vi "Main.vi"() -> ()   [LabVIEW 2013]
uses:
  <vilib>/event_ctls.llb/eventvkey.ctl
  skripte/Element 1.ctl
  Global_Not-Aus.vi
  <vilib>/Utility/file.llb/Read From Spreadsheet File (DBL).vi
  Global_Start_Stop_Einzelschritt.vi
  <vilib>/Utility/file.llb/Write To Spreadsheet File (DBL).vi
  <vilib>/Utility/file.llb/Read From Spreadsheet File (string).vi
  <vilib>/Utility/file.llb/Write To Spreadsheet File (string).vi
  <vilib>/Instr/_visa.llb/VISA Configure Serial Port (Instr).vi
panel:
  out "temp":string
  in  "stop handover":bool
  in  "Polplan":string[](array[string])
  in  "load polplan":bool
  in  "Second head On/Off":bool
  in  "path polplan":path
  in  "distance measure mode":string(combo)="ED33"
  in  "start auto write":bool
  out "key stm 2":string
  in  "baud rate (9600) 4":u32=921600 caption="Baudrate (9600)"
  in  "baud rate (9600) 3":u32=19200 caption="Baudrate (9600)"
  in  "string to write 2":string="?MEAS\r" caption="Zu schreibender String"
  out "read string 8":string caption="Gelesener String"
  out "read string 7":string caption="Gelesener String"
  in  "delay before read (ms) 7":u32=300 caption="Verzögerung vor dem Lesen (ms)"
  out "Mess Zähler":dbl
  in  "Boolesch1 25":bool
  in  "Pfad 2":path
  in  "path Selection":T1(ring)
  in  "Boolesch1 24":bool
  in  "Boolesch1 23":bool
  in  "Boolesch1 22":bool
  in  "Boolesch1 21":bool
  in  "Boolesch1 20":bool
  in  "Boolesch1 19":bool
  in  "Boolesch1 18":bool
  in  "Boolesch1 17":bool
  in  "Boolesch1 16":bool
  in  "Boolesch1":bool
  in  "Boolesch1 15":bool
  in  "Boolesch1 14":bool
  in  "Boolesch1 13":bool
  in  "Boolesch1":bool
  in  "Boolesch1 12":bool
  in  "Boolesch1 11":bool
  in  "Boolesch1 3":bool
  in  "Boolesch1 2":bool
  in  "Boolesch1":bool
  in  "Boolesch1":bool
  in  "Pfad 20":path
  in  "Pfad 19":path
  in  "Pfad 18":path
  in  "Pfad 17":path
  in  "Pfad 16":path
  in  "Pfad 15":path
  in  "Pfad 14":path
  in  "Pfad 13":path
  in  "Pfad 12":path
  in  "Pfad 11":path
  in  "Pfad 10":path
  in  "Pfad 9":path
  in  "Pfad 8":path
  in  "Pfad 7":path
  in  "Pfad 6":path
  in  "Pfad 5":path
  in  "Pfad 4":path
  in  "Pfad2":path
  in  "Pfad 0":path
  out "Messsensor":string
  out "key stm 5":string
  out "key stm 4":string
  out "key stm 3":string
  in  "baud rate 6":u32=921600 caption="Baudrate"
  in  "data bits 6":u16=8 caption="Datenbits" min=5 max=8 step=1
  in  "parity 6":u16(ring) caption="Parität" items=["Keine", "Ungerade", "Gerade", "Mark", "Space"]
  in  "stop bits 6":u16(ring)=10 caption="Stoppbits" items=["1.0"=10, "1.5"=15, "2.0"=20]
  in  "flow control 6":u16(ring) caption="Ablaufsteuerung" items=["Keine"=0, "XON/XOFF"=1, "RTS/CTS"=2, "DTR/DSR"=4]
  in  "baud rate (9600) 2":u32=115200 caption="Baudrate (9600)"
  in  "delay before read (ms) 6":u32=100 caption="Verzögerung vor dem Lesen (ms)"
  in  "write ED33":string="?\r" caption="Remote_Modus"
  out "bytes read 6":u32 caption="Gelesene Bytes"
  out "read string 6":string caption="Gelesener String2"
  in  "write KMT":string="o\r" caption="Remote_Modus"
  out "read string 5":string caption="Gelesener String"
  in  "Start ED33 schreiben":bool
  out "read string 4":string caption="Gelesener String"
  out "bytes read 5":u32 caption="Gelesene Bytes"
  in  "write 10":string="Z\r" caption="Remote_Modus"
  in  "delay before read (ms) 5":u32=100 caption="Verzögerung vor dem Lesen (ms)"
  in  "write 9":bool=TRUE caption="Schreiben"
  in  "flow control 5":u16(ring) caption="Ablaufsteuerung" items=["Keine"=0, "XON/XOFF"=1, "RTS/CTS"=2, "DTR/DSR"=4]
  in  "stop bits 5":u16(ring)=10 caption="Stoppbits" items=["1.0"=10, "1.5"=15, "2.0"=20]
  in  "parity 5":u16(ring) caption="Parität" items=["Keine", "Ungerade", "Gerade", "Mark", "Space"]
  in  "data bits 5":u16=8 caption="Datenbits" min=5 max=8 step=1
  in  "VISA-Referenz (Eingang) 3":refnum<visa-resource-name>="COM7" caption="VISA-Ressourcenname"
  in  "baud rate 5":u32=921600 caption="Baudrate"
  out "bytes read 4":u32 caption="Gelesene Bytes"
  in  "write9":string="Z\r" caption="Remote_Modus"
  in  "delay before read (ms) 4":u32=100 caption="Verzögerung vor dem Lesen (ms)"
  in  "write 8":bool=TRUE caption="Schreiben"
  in  "flow control 4":u16(ring) caption="Ablaufsteuerung" items=["Keine"=0, "XON/XOFF"=1, "RTS/CTS"=2, "DTR/DSR"=4]
  in  "stop bits 4":u16(ring)=10 caption="Stoppbits" items=["1.0"=10, "1.5"=15, "2.0"=20]
  in  "parity 4":u16(ring) caption="Parität" items=["Keine", "Ungerade", "Gerade", "Mark", "Space"]
  in  "data bits 4":u16=8 caption="Datenbits" min=5 max=8 step=1
  in  "VISA-Referenz (Eingang) 2":refnum<visa-resource-name>="COM7" caption="VISA-Ressourcenname"
  in  "baud rate 4":u32=921600 caption="Baudrate"
  out "Position Y ED33 2":string
  out "bytes read 3":u32 caption="Gelesene Bytes"
  in  "write 7":string="?\r" caption="Remote_Modus"
  in  "delay before read (ms) 3":u32=100 caption="Verzögerung vor dem Lesen (ms)"
  in  "write 6":bool=TRUE caption="Schreiben"
  in  "flow control 3":u16(ring) caption="Ablaufsteuerung" items=["Keine"=0, "XON/XOFF"=1, "RTS/CTS"=2, "DTR/DSR"=4]
  in  "stop bits 3":u16(ring)=10 caption="Stoppbits" items=["1.0"=10, "1.5"=15, "2.0"=20]
  in  "parity 3":u16(ring) caption="Parität" items=["Keine", "Ungerade", "Gerade", "Mark", "Space"]
  in  "data bits 3":u16=8 caption="Datenbits" min=5 max=8 step=1
  in  "VISA-Referenz (Eingang)":refnum<visa-resource-name>="COM7" caption="VISA-Ressourcenname"
  in  "baud rate 3":u32=921600 caption="Baudrate"
  out "Position Y ED33":string
  out "read string 3":string caption="Gelesener String"
  out "bytes read 2":u32 caption="Gelesene Bytes"
  in  "delay before read (ms) 2":u32=100 caption="Verzögerung vor dem Lesen (ms)"
  in  "write 4":bool=TRUE caption="Schreiben"
  in  "flow control 2":u16(ring) caption="Ablaufsteuerung" items=["Keine"=0, "XON/XOFF"=1, "RTS/CTS"=2, "DTR/DSR"=4]
  in  "stop bits 2":u16(ring)=10 caption="Stoppbits" items=["1.0"=10, "1.5"=15, "2.0"=20]
  in  "parity 2":u16(ring) caption="Parität" items=["Keine", "Ungerade", "Gerade", "Mark", "Space"]
  in  "data bits 2":u16=8 caption="Datenbits" min=5 max=8 step=1
  in  "baud rate 2":u32=921600 caption="Baudrate"
  in  "delay before read (ms)":u32=100 caption="Verzögerung vor dem Lesen (ms)"
  in  "write 3":string="?\r" caption="Remote_Modus"
  out "bytes read":u32 caption="Gelesene Bytes"
  out "Serial Settings:Number of Bytes at Serial Port":u32
  out "read string 2":string caption="Gelesener String2"
  in  "write 2":string="os\r" caption="Remote_Modus"
  out "read string":string caption="Gelesener String"
  in  "baud rate (9600)":u32=115200 caption="Baudrate (9600)"
  in  "flow control":u16(ring) caption="Ablaufsteuerung" items=["Keine"=0, "XON/XOFF"=1, "RTS/CTS"=2, "DTR/DSR"=4]
  in  "stop bits":u16(ring)=10 caption="Stoppbits" items=["1.0"=10, "1.5"=15, "2.0"=20]
  in  "parity":u16(ring) caption="Parität" items=["Keine", "Ungerade", "Gerade", "Mark", "Space"]
  in  "data bits":u16=8 caption="Datenbits" min=5 max=8 step=1
  in  "baud rate":u32=921600 caption="Baudrate"
  in  "Normal Betrieb":bool
  in  "Standard memory":T2={"mm Xmin "=0.0, "mm Xmax "=100.0, " mm Ymin "=0.0, "mm Ymax "=267.9, " mm Zmin"=0.0, "mm Zmax "=108.0, "Schritte oder mm Umin (0)"=0.0, "Schritte oder mm Umax (0)"=0.0, "Schritte oder mm Cmin (0)"=0.0, "Schritte oder mm Cmax (0)"=0.0, "Schritte oder mm Amin (0)"=0.0, "Schritte oder mm Amax (0)"=0.0, "Schritte oder mm Bmin (0)"=0.0, "Schritte oder mm Bmax (0)"=0.0}
  in  "save reference kmt":bool
  in  "go to reference kmt":bool
  in  "set reference KMT":bool
  out "Referenz KMT":dbl[](array[numeric])
  out "current sequence":string[](array[string])
  in  "sequence active?":bool
  in  "clear sequence":bool
  in  "Load sequence":bool
  in  "Pfad 1":path
  out "sequence":string[][](array[string])
  in  "save reference head":bool
  in  "go to reference head":bool
  in  "set reference head":bool
  out "Reference Write head":dbl[](array[numeric])
  out "KMT Output":string
  out "STM run":dbl
  out "Write head Output":string
  in  "Power Supply Init":T3(tab)
  in  "go relative":T4
  in  "straight absolute":bool
  in  "go to exchange position":bool
  in  "read":bool
  in  "set speed btn":bool
  in  "set speed":dbl caption="[mm/s]"
  in  "go straight relative":bool
  in  "magnetization set":bool
  in  "magnetization":u16(ring) items=["off", "positive", "negative"]
  in  "command list":string(combo)
  in  "manual control OK":bool
  in  "coordinates":dbl[](array[numeric])
  in  "Absolute":bool
  out "KMT read":bool
  in  "Distances":T5
  in  "Direction 2":T6 {"Richtung Z (vEw)" items=["vom Endschalter weg", "zum Endschalter hin"]; "Richtung Y (vEw)" items=["vom Endschalter weg", "zum Endschalter hin"]; "Richtung X (vEw)" items=["vom Endschalter weg", "zum Endschalter hin"]}
  out "Measurement start value":T7
  in  "Movement":dbl[](array[numeric])
  out "ED33reading":bool
  out "GAUS read":bool
  in  "p10":dbl[](array[numeric])
  in  "p9":dbl[](array[numeric])
  in  "p8":dbl[](array[numeric])
  in  "p7":dbl[](array[numeric])
  in  "p6":dbl[](array[numeric])
  in  "p5":dbl[](array[numeric])
  in  "p4":dbl[](array[numeric])
  in  "p3":dbl[](array[numeric])
  in  "p2":dbl[](array[numeric])
  in  "Enum":T8(ring)
  in  "p1":dbl[](array[numeric])
  in  "speichern":bool
  in  "Batch field memory":path=path "Y:/01_Projekte/EPN93031_Schreibplatz/8_Konstruktionsunterlagen/8.5_Software/KOSY Steuerung LabVIEW/Batch_position1" caption="Dateipfad (Dialog, wenn leer)"
  in  "Als Standart":bool
  in  "bo to batch":bool
  in  "Enum 2":T9(ring)
  out "sensor log":string[][](table)
  in  "clear sensor log":bool
  in  "sequence path":path
  in  "open Log":bool
  in  "save log":bool
  out "XY Graph":cluster{"Y":dbl[], "Y":dbl[]}[](graph) caption="XY-Graph"
  in  "Plot":u16(ring)=6 items=["Sinus1"=5, "Cosinus1"=6, "Sinus2"=7, "Cosinus2"=8]
  out "Array":string[](array[string])
  in  "sensor run constant read":bool
  out "error IO":errorcluster caption="Error In"
  out "log":string
  out "movement":T10={"Achsen-Wahl (X)"=36, "Richtung (vEw)"=0, "Geschwindigkeit\nin mm/s (5)[0,025-20]"=5.0, "IV6"=FALSE} {"Richtung (vEw)" items=["vom Endschalter weg", "zum Endschalter hin"]; "Geschwindigkeit\nin mm/s (5)[0,025-20]" min=0.025 max=20; "Achsen-Wahl (X)" items=["X-Achse"=36, "Y-Achse"=37, "Z-Achse"=38, "U-Achse"=63]}
  out "key":T12
  in  "Anwenden":bool
  in  "Set as new standard":bool
  in  "Standartwiderherstellen Bereiche":bool
  out "Power supply init":string[](array[string])
  in  "Bereiche  X,Y,Z":T2={"mm Xmin "=0.0, "mm Xmax "=100.0, " mm Ymin "=0.0, "mm Ymax "=267.9, " mm Zmin"=0.0, "mm Zmax "=108.0, "Schritte oder mm Umin (0)"=0.0, "Schritte oder mm Umax (0)"=0.0, "Schritte oder mm Cmin (0)"=0.0, "Schritte oder mm Cmax (0)"=0.0, "Schritte oder mm Amin (0)"=0.0, "Schritte oder mm Amax (0)"=0.0, "Schritte oder mm Bmin (0)"=0.0, "Schritte oder mm Bmax (0)"=0.0}
  in  "Choose file spaces":path=path "Y:/01_Projekte/EPN93031_Schreibplatz/8_Konstruktionsunterlagen/8.5_Software/KOSY Steuerung LabVIEW/Bereichsref"
  in  "Port KOSY":refnum<visa-resource-name>="COM2"
  in  "Port ED32i":refnum<visa-resource-name>="COM8"
  in  "Port ED33":refnum<visa-resource-name>="COM7"
  in  "Port Write head":refnum<visa-resource-name>="COM4"
  in  "Port Netzteil":refnum<visa-resource-name>="COM3" caption="Port Power Supply"
  in  "KMT Port":refnum<visa-resource-name>="COM11" caption="Port KMT"
  in  "GAUS Port":refnum<visa-resource-name>="COM5" caption="Port GAUS"
  in  "GAUS read strart 2":bool
  in  "Save as text":bool
  out "Attached Array":string[][](array[string])
  in  "ED 33 Start":bool
  in  "write 5":string="z\r" caption="ED33 reset"
  in  "KMT read start":bool
  in  "Path to save txt files":path=path "Y:/01_Projekte/EPN93031_Schreibplatz/8_Konstruktionsunterlagen/8.5_Software/KOSY Steuerung LabVIEW/Messdaten Speicher"
  in  "stop program":bool
  out "moving":bool
  out "Stopped":bool
  out "current coordinates":T7
  out "speed":dbl(knob) scale=0.0..20.0
  out "key stm":string
  out "cancel state":string
  # "adress  ADR 00"
  # "remote mode"
  # "Set voltage to 10 V"
  # "Set  current to 1 A"
  # "adress  ADR 01"
  # "remote mode"
  # "Set voltage to 10 V"
  # "Set  current to 1 A"
  # "Sensors"
  # "power supply"
  # "KOSY"
types:
  T1 = enum16{"0", "1", "2", "3", "4", "5", "6", "7", "8", "9", "10", "11", "12", "13", "14", "15", "16", "17", "18", "19", "20", ""}
  T2 = cluster{"mm Xmin ":sgl, "mm Xmax ":sgl, " mm Ymin ":sgl, "mm Ymax ":sgl, " mm Zmin":sgl, "mm Zmax ":sgl, "Schritte oder mm Umin (0)":sgl, "Schritte oder mm Umax (0)":sgl, "Schritte oder mm Cmin (0)":sgl, "Schritte oder mm Cmax (0)":sgl, "Schritte oder mm Amin (0)":sgl, "Schritte oder mm Amax (0)":sgl, "Schritte oder mm Bmin (0)":sgl, "Schritte oder mm Bmax (0)":sgl}
  T3 = enum32{"manual control", "Polstreifen", "MeasuringField", "BatchField", "sensor log", "Sensorfahrt", "debug", "Info", "settings", "sensor log 2"}
  T4 = typedef "Element 1.ctl" = bool
  T5 = cluster{"X-Abstand (0)":sgl, "Y-Abstand (0)":sgl, "Z-Abstand (0)":sgl}
  T6 = cluster{"Richtung X (vEw)":u16, "Richtung Y (vEw)":u16, "Richtung Z (vEw)":u16}
  T7 = cluster{"steps x":dbl, "steps y":dbl, "steps z":dbl, "steps u":dbl, "steps c":dbl, "steps a":dbl, "steps b":dbl}
  T8 = enum16{"Position 1", "Position 2", "Position 3", "Position 4", "Position 5", "Position 6", "Position 7", "Position 8", "Position 9", "Position 10"}
  T9 = enum16{"p1", "p2", "p3", "p4", "p5", "p6", "p7", "p8", "p9", "p10"}
  T10 = cluster{"Achsen-Wahl (X)":u8, "Richtung (vEw)":u8, "Geschwindigkeit\nin mm/s (5)[0,025-20]":sgl, "IV6":bool}
  T11 = typedef "eventvkey.ctl" = enum16{"ASCII", "Enter", "Return", "Shift", "Ctrl", "Alt", "Cmd", "Opt", "Caps", "NumLock", "Clear", "Break", "Up", "Down", "Left", "Right", "Insert", "Delete", "Home", "End", "PageUp", "PageDown", "Escape", "Help", "Pause", "ScrollLock", "F1", "F2", "F3", "F4", "F5", "F6", "F7", "F8", "F9", "F10", "F11", "F12", "F13", "F14", "F15", "F16", "F17", "F18", "F19", "F20", "F21", "F22", "F23", "F24", "Play", "VolumeUp", "VolumeDown", "Mute", "Two Byte Char"}
  T12 = cluster{"laufende Nummer":i16, "Vkey":T11, "Taste":i32}
  T13 = enum16{"vom Endschalter weg", "zum Endschalter hin"}
  T14 = enum16{"zum Endschalter hin", "vom Endschalter weg"}
  T15 = cluster{"[0]":sgl, "[1]":sgl, "[2]":sgl, "[3]":sgl, "[4]":sgl, "[5]":sgl, "[6]":sgl, "[7]":sgl, "[8]":sgl, "[9]":sgl, "[10]":sgl, "[11]":sgl, "[12]":sgl, "[13]":sgl}
  T16 = cluster{"Schritte X":sgl, "Schritte Y":sgl, "Schritte Z":sgl, "Schritte U":sgl, "Schritte C":sgl, "Schritte A":sgl, "Schritte B":sgl}
  T17 = cluster{"Element":dbl, "Element":dbl, "Element":dbl}
  T18 = cluster{"coordinates[0]":dbl, "coordinates[1]":dbl, "coordinates[2]":dbl, "coordinates[3]":dbl, "coordinates[4]":dbl, "coordinates[5]":dbl, "coordinates[6]":dbl, "coordinates[7]":dbl, "coordinates[8]":dbl}
  T19 = cluster{u16, enum16{"vom Endschalter weg", "zum Endschalter hin"}, enum16{"vom Endschalter weg", "zum Endschalter hin"}}
  T20 = cluster{"coordinates[0]":dbl, "coordinates[1]":dbl, "coordinates[2]":dbl}
  T21 = cluster{"[0]":dbl, "[1]":dbl, "[2]":dbl, "[3]":dbl, "[4]":dbl, "[5]":dbl, "[6]":dbl, "[7]":dbl, "[8]":dbl}
  T22 = cluster{"Movement[0]":dbl, "Movement[1]":dbl, "Movement[2]":dbl, "Movement[3]":dbl, "Movement[4]":dbl, "Movement[5]":dbl, "Movement[6]":dbl, "Movement[7]":dbl, "Movement[8]":dbl}
  T23 = cluster{"Movement[0]":dbl, "Movement[1]":dbl, "Movement[2]":dbl, "X-Abstand (0)":sgl, "Y-Abstand (0)":sgl, "Z-Abstand (0)":sgl, "Movement[6]":dbl, "Movement[7]":dbl, "Movement[8]":dbl}
  T24 = cluster{"[0]":string, "[1]":string, "[2]":string, "[3]":string, "[4]":string, "[5]":string, "[6]":string, "[7]":string, "[8]":string}
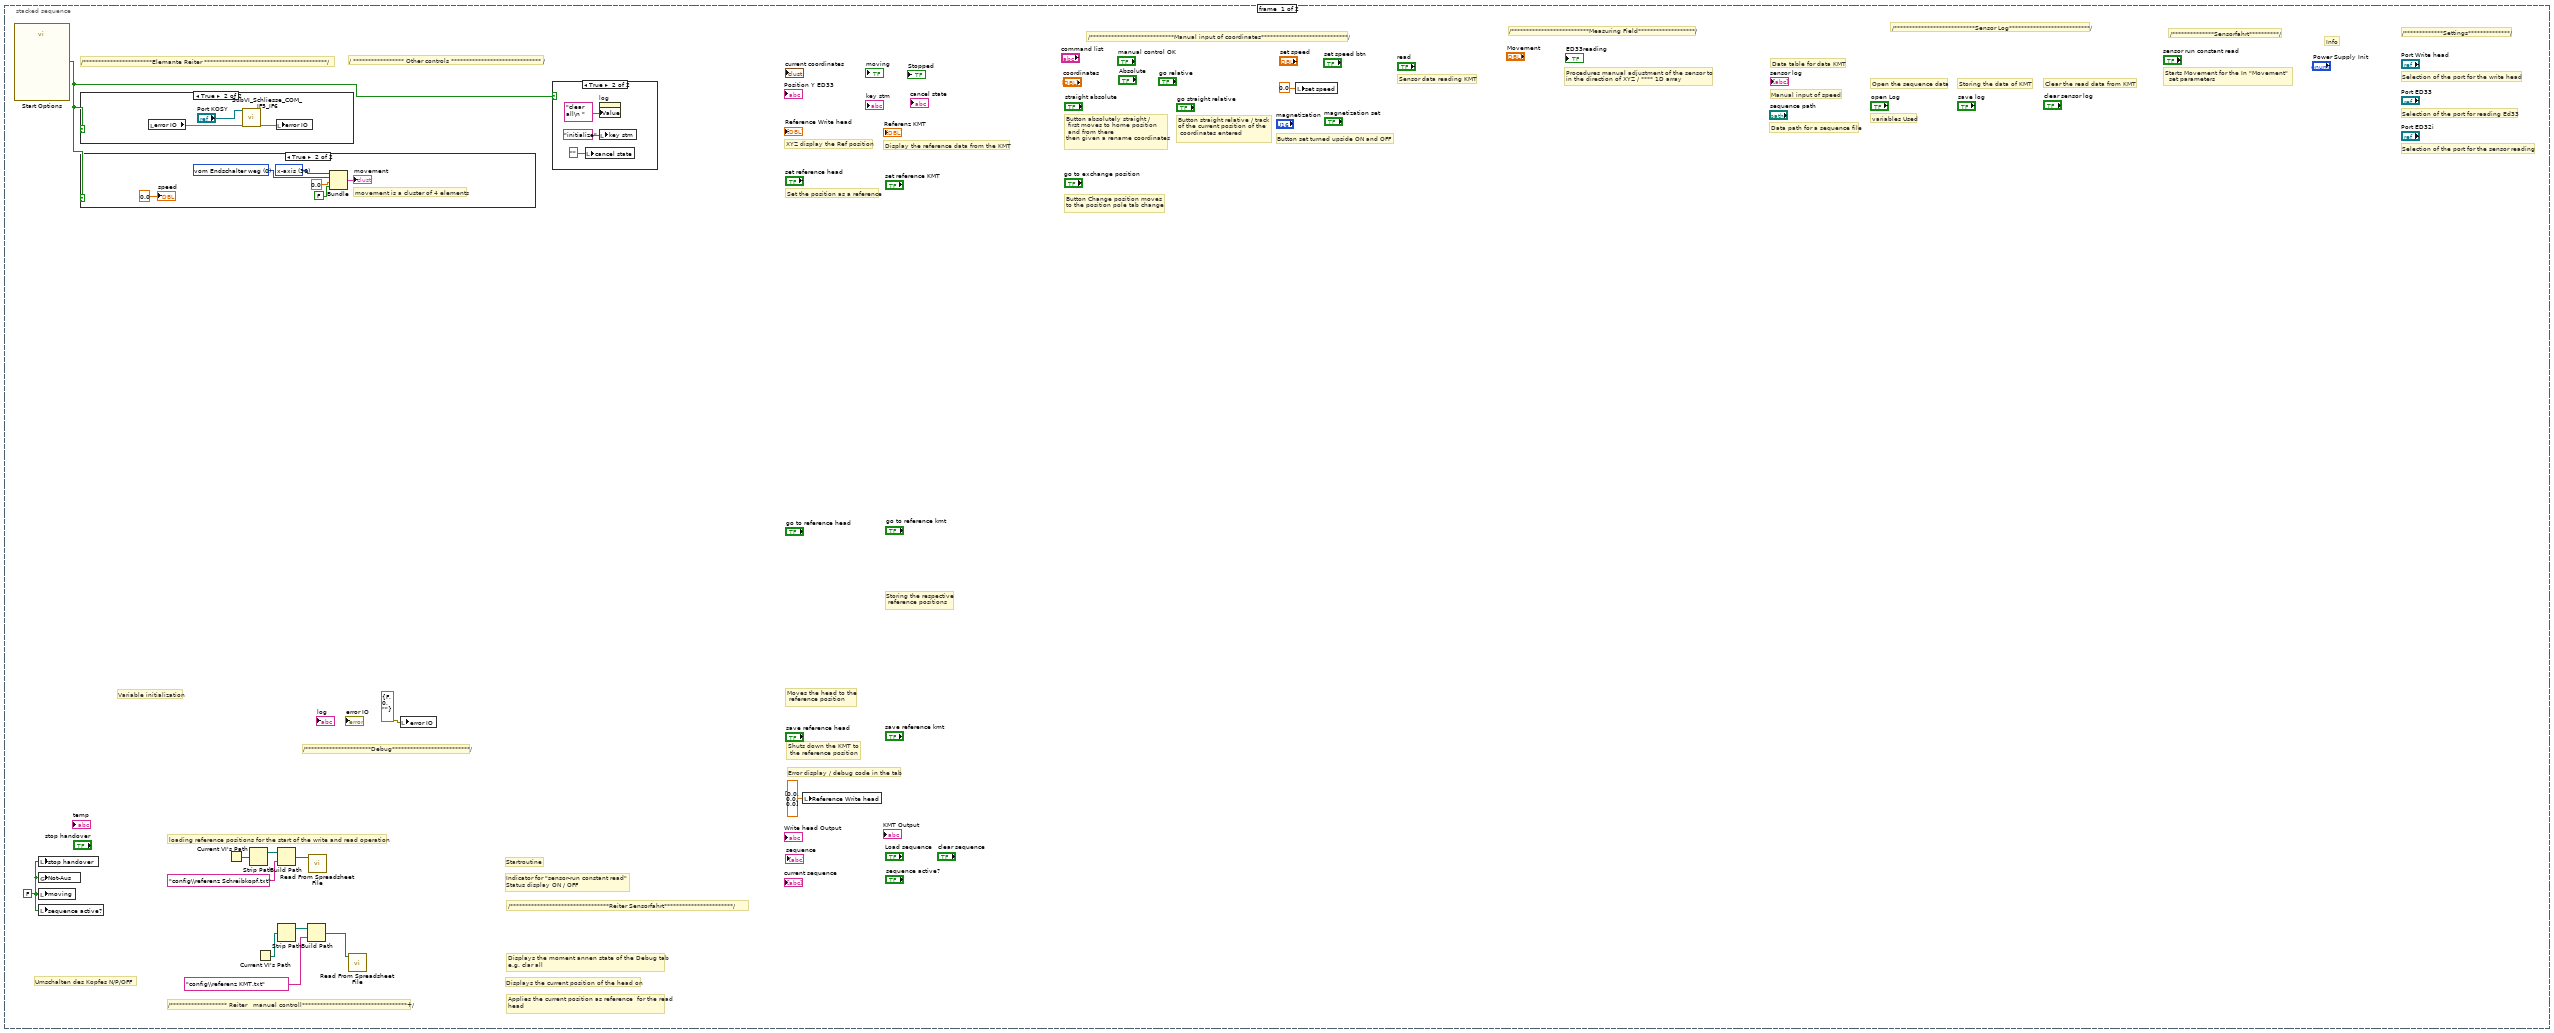
[diagram p2: hidden frame]
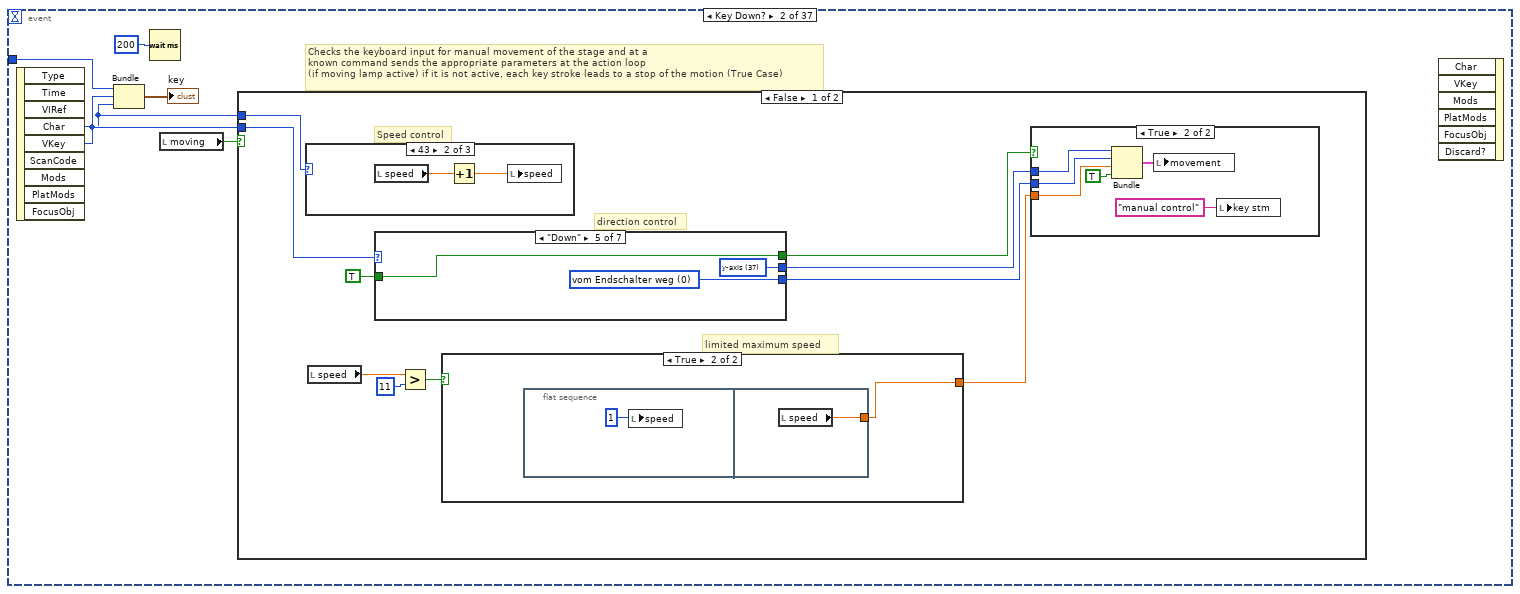
[diagram p6: hidden frame]
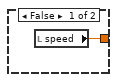
[diagram p7: hidden frame]
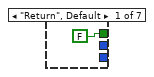
[diagram p9: hidden frame]
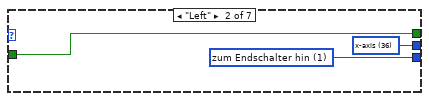
[diagram p10: hidden frame]
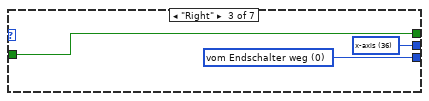
[diagram p11: hidden frame]
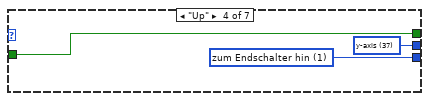
[diagram p12: hidden frame]
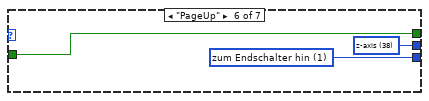
[diagram p13: hidden frame]
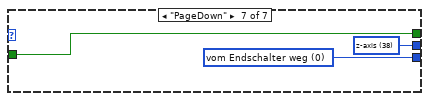
[diagram p14: hidden frame]
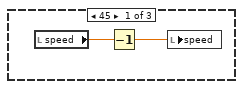
[diagram p15: hidden frame]
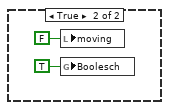
[diagram p17: hidden frame]
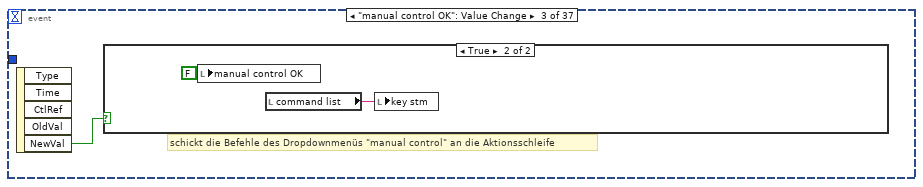
[diagram p18: hidden frame]
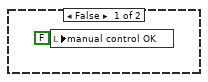
[diagram p19: hidden frame]
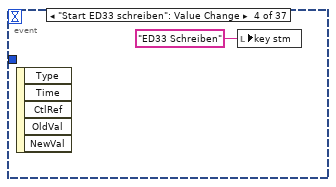
[diagram p20: hidden frame]
diagram:
  n1 = stacked-sequence {
    tunnel: [_ w27] -> w1
    frame #0 {
      w12 = FALSE
      # "/*************Settings**************/"
      # "Info"
      # "/**********************Debug**************************/"
      # "/**************Sensorfahrt**********/"
      # "/***************************Sensor Log***************************/"
      # "/**************************Measuring Field*******************/"
      # "Applies the current position as reference  for the read head"
      # "Indicator for \"sensor-run constant read\"\nStatus display ON / OFF"
      # "/*********************************Reiter Sensorfahrt***********************/"
      # "Displays the moment annen state of the Debug tab\ne.g. clar all"
      # "Selection of the port for the write head"
      # "XYZ display the Ref position"
      # "Set the position as a reference"
      # "Storing the respective\n reference positions"
      # "Open the sequence data"
      # "Storing the data of KMT"
      # "Shuts down the KMT to\n the reference position"
      # "Moves the head to the\n reference position"
      # "Data path for a sequence file"
      # "Display the reference data from the KMT"
      # "Selection of the port for reading Ed33"
      # "Sensor data reading KMT"
      # "Data table for data KMT"
      # "Clear the read data from KMT"
      # "Selection of the port for the sensor reading"
      # "Displays the current position of the head on"
      # "/ ***************** Other controls ****************************** /"
      # "Manual input of speed"
      # "Button straight relative / track \nof the current position of the\n coordinates entered"
      # "Umschalten des Kopfes N/P/OFF"
      # "Button set turned upside ON and OFF"
      # "Button absolutely straight /\n first moves to home position\n and from there\nthen given a rename coordinates"
      # "Button Change position moves \nto the position pole tab change"
      # "/****************************Manual input of coordinates*****************************/"
      # "/******************* Reiter   manuel controll***********************************+/"
      # "Starts Movement for the In \"Movement\"\n  set parameters"
      # "Procedures manual adjustment of the sensor to\nin the direction of XYZ / **** 1D array"
      # "/***********************Elemante Reiter *****************************************/"
      # "Error display / debug code in the tab"
      # "loading reference positions for the start of the write and read operation"
      # "Variable initialization"
      # "variables Used"
      # "Startroutine"
      n2 = call "Start Options"() -> ("Initialize"=w13:bool)  [unwired: 18 in, 1 out]
      n3 = local write "stop handover"(w12) -> ()
      n4 = global write "Global_Not-Aus.vi" "Not-Aus"(w12) -> ()
      n5 = local write "moving"(w12) -> ()
      n6 = local write "sequence active?"(w12) -> ()
      n7 = case shown="True" w13 {
        frame False {
        }
        frame True {
          n8 = local read "error IO"() -> (w25:errorcluster)
          n9 = call "SubVI_Schliesse_COM_IF5_IF6.vi"("VISA resource name in"="Port KOSY", "error in"=w25) -> ("error out"=w24:errorcluster)  [unwired: 13 in]
          n10 = local write "error IO"(w24) -> ()
        }
      }
      n11 = case shown="True" w13 {
        frame False {
        }
        frame True {
          w18 = u16 0 items=["vom Endschalter weg", "zum Endschalter hin"]
          w19 = u16 36 items=["x-axis"=36, "y-axis"=37, "z-axis"=38]
          # "movement is a cluster of 4 elements"
          n12 = Bundle(w19, w18, 0.0, FALSE) -> (→"movement":cluster{u16, u16, dbl, bool})  [unwired: 1 in]
          "speed" <- 0.0
        }
      }
      n13 = Current VI's Path() -> (path=w8:path)
      n14 = Strip Path(path=w8) -> (stripped path=w7:path)  [unwired: 1 out]
      n15 = Current VI's Path() -> (path=w5:path)
      n16 = Build Path(base path=w7, name or relative path="config\\referenz Schreibkopf.txt") -> (appended path=w3:path)
      n17 = Strip Path(path=w5) -> (stripped path=w4:path)  [unwired: 1 out]
      n18 = Build Path(base path=w4, name or relative path="config\\referenz KMT.txt") -> (appended path=w2:path)
      n19 = call-poly <vilib>:"Read From Spreadsheet File.vi"("file path (dialog if empty)"=w3) -> ()  [unwired: 6 in, 5 out]
      n20 = call-poly <vilib>:"Read From Spreadsheet File.vi"("file path (dialog if empty)"=w2) -> ()  [unwired: 6 in, 5 out]
      n21 = local write "error IO"(errorcluster {"status"=FALSE, "code"=0, "source"=""} ("error IO")) -> ()
      n22 = case shown="True" w13 {
        frame False {
        }
        frame True {
          n23 = local write "cancel state"("") -> ()
          n24 = property on="log" class="Str"("Value"="clear all\n " ("Zustand")) -> ()  [unwired: 2 in, 2 out]
          n25 = local write "key stm"("initialize") -> ()
        }
      }
      n26 = local write "Reference Write head"(dbl[] [0.0, 0.0, 0.0]) -> ()
      n27 = local write "set speed"(0.0) -> ()
    }
    frame #1 {
      # "Loop in which all commands are translated into action"
      # "While loop, the events (key presses or\nButtons) intercepts and the corresponding command to the\nAction loop forwards."
      n28 = while {
        i -> [w44]
        stop <- w43 stop-if-true
        # "constant updating of the graph, which records the results of the sensor logs"
        n29 = event shown="[0] Timeout" {
          selector: _ -> [_ _ _ _ _ _ _ _ _ _ _ _ _ _ _ _ _ _ _ _ _ _ _ _ _ _ _ _ _ _ _ _ _ _ _ _ _]
          dyn-events: _ -> [_ _ _ _ _ _ _ _ _ _ _ _ _ _ _ _ _ _ _ _ _ _ _ _ _ _ _ _ _ _ _ _ _ _ _ _ _]
          timeout: 50 -> [_ _ _ _ _ _ _ _ _ _ _ _ _ _ _ _ _ _ _ _ _ _ _ _ _ _ _ _ _ _ _ _ _ _ _ _ _]
          tunnel: w44 -> [_ w51 _ _ _ _ _ _ _ _ _ _ _ _ _ _ _ _ _ _ _ _ _ _ _ _ _ _ _ _ _ _ _ _ _ _ _]
          event Timeout {
            n30 = event-data() -> ()  [unwired: 1 in, 2 out]
            n31 = global write "Global_Start_Stop_Einzelschritt.vi" "Boolesch"(FALSE) -> ()
          }
          event Key Down? {
            # "Checks the keyboard input for manual movement of the stage and at a \nknown command sends the appropriate parameters at the action loop \n(if moving lamp active) if it is not active, each key stroke leads to a stop of the motion (True Case)"
            n32 = event-data() -> ("Char"=w46:i16, "VKey"=w49:T11)  [unwired: 1 in, 7 out]
            n33 = Bundle(w51, "VKey"=w49, "Char"=w46) -> (→"key":cluster{i32, "VKey":T11, "Char":i16})  [unwired: 1 in]
            n34 = Wait (ms)(milliseconds to wait=200) -> ()  [unwired: 1 out]
            n35 = local read "moving"() -> (w48:bool)
            n36 = case shown="False" w48 {
              tunnel: w49 -> [w61 _]
              tunnel: w46 -> [w57 _]
              frame False {
                # "direction control"
                # "Speed control"
                # "limited maximum speed"
                n37 = case "Case-Struktur" shown="43" w57 {
                  frame 45 {
                    n38 = local read "speed"() -> (w92:dbl)
                    n39 = Decrement(x=w92) -> (x-1=w91:dbl)
                    n40 = local write "speed"(w91) -> ()
                  }
                  frame 43 {
                    n41 = local read "speed"() -> (w93:dbl)
                    n42 = Increment(x=w93) -> (x+1=w94:dbl)
                    n43 = local write "speed"(w94) -> ()
                  }
                  frame 55, Default {
                  }
                }
                n44 = local read "speed"() -> (w56:dbl)
                n45 = case shown="\"Down\"" w61 {
                  tunnel: [FALSE w75 w78 w81 w84 w87 w90] -> w52
                  tunnel: TRUE -> [_ w75 w78 w81 w84 w87 w90]
                  tunnel: [_ w74 w77 w80 w83 w86 w89] -> w59
                  tunnel: [_ w73 w76 w79 w82 w85 w88] -> w58
                  frame "Return", Default {
                  }
                  frame "Left" {
                    w73 = u16 1 items=["vom Endschalter weg", "zum Endschalter hin"]
                    w74 = u16 36 items=["x-axis"=36, "y-axis"=37, "z-axis"=38]
                  }
                  frame "Right" {
                    w76 = u16 0 items=["vom Endschalter weg", "zum Endschalter hin"]
                    w77 = u16 36 items=["x-axis"=36, "y-axis"=37, "z-axis"=38]
                  }
                  frame "Up" {
                    w79 = u16 1 items=["vom Endschalter weg", "zum Endschalter hin"]
                    w80 = u16 37 items=["x-axis"=36, "y-axis"=37, "z-axis"=38]
                  }
                  frame "Down" {
                    w82 = u16 0 items=["vom Endschalter weg", "zum Endschalter hin"]
                    w83 = u16 37 items=["x-axis"=36, "y-axis"=37, "z-axis"=38]
                  }
                  frame "PageUp" {
                    w85 = u16 1 items=["vom Endschalter weg", "zum Endschalter hin"]
                    w86 = u16 38 items=["x-axis"=36, "y-axis"=37, "z-axis"=38]
                  }
                  frame "PageDown" {
                    w88 = u16 0 items=["vom Endschalter weg", "zum Endschalter hin"]
                    w89 = u16 38 items=["x-axis"=36, "y-axis"=37, "z-axis"=38]
                  }
                }
                n46 = Greater?(x=w56, y=11) -> (0:w54:bool)
                n47 = case shown="True" w54 {
                  tunnel: [w62 w63] -> w53
                  frame False {
                    n48 = local read "speed"() -> (w62:dbl)
                  }
                  frame True {
                    n49 = flat-sequence {
                      tunnel: [w65] -> w63
                      frame #0 {
                        n50 = local write "speed"(1) -> ()
                      }
                      frame #1 {
                        n51 = local read "speed"() -> (w65:dbl)
                      }
                    }
                  }
                }
                n52 = case shown="True" w52 {
                  tunnel: w59 -> [_ w71]
                  tunnel: w58 -> [_ w70]
                  tunnel: w53 -> [_ w66]
                  frame False {
                  }
                  frame True {
                    n53 = Bundle(w71, w70, "speed"=w66, TRUE) -> (w68:cluster{u16, u16, "speed":dbl, bool})  [unwired: 1 in]
                    n54 = local write "movement"(w68) -> ()
                    n55 = local write "key stm"("manual control") -> ()
                  }
                }
              }
              frame True {
                n56 = local write "moving"(FALSE) -> ()
                n57 = global write "Global_Start_Stop_Einzelschritt.vi" "Boolesch"(TRUE) -> ()
              }
            }
            n58 = event-data() -> ()  [unwired: 7 in, 1 out]
          }
          event "manual control OK": Value Change {
            # "schickt die Befehle des Dropdownmenüs \"manual control\" an die Aktionsschleife"
            n59 = event-data() -> ("NewVal"=w97:bool)  [unwired: 1 in, 4 out]
            n60 = case shown="True" w97 {
              frame False {
                n61 = local write "manual control OK"(FALSE) -> ()
              }
              frame True {
                n62 = local write "manual control OK"(FALSE) -> ()
                n63 = local read "command list"() -> (w100:string)
                n64 = local write "key stm"(w100) -> ()
              }
            }
          }
          event "Start ED33 schreiben": Value Change {
            n65 = event-data() -> ()  [unwired: 1 in, 5 out]
            n66 = local write "key stm"("ED33 Schreiben" ("key stm")) -> ()
          }
          event "Absolute": Value Change {
            n67 = event-data() -> ("NewVal"=w102:bool)  [unwired: 1 in, 4 out]
            n68 = case shown="True" w102 {
              frame False {
              }
              frame True {
                n69 = local write "Absolute"(FALSE) -> ()
                n70 = local write "key stm"("go to coordinates") -> ()
              }
            }
          }
          event "straight absolute": Value Change {
            n71 = event-data() -> ("NewVal"=w105:bool)  [unwired: 1 in, 4 out]
            n72 = case shown="True" w105 {
              frame False {
              }
              frame True {
                n73 = local write "straight absolute"(FALSE) -> ()
                n74 = local write "key stm"("go straight to coordinates") -> ()
              }
            }
          }
          event Value Change {
            n75 = event-data() -> ("NewVal"=w108:T4)  [unwired: 1 in, 4 out]
            n76 = case shown="True" w108 {
              frame False {
              }
              frame True {
                n77 = local write "go relative"(FALSE) -> ()
                n78 = local write "key stm"("go relative") -> ()
              }
            }
          }
          event "go straight relative": Value Change {
            n79 = event-data() -> ("NewVal"=w111:bool)  [unwired: 1 in, 4 out]
            n80 = case shown="True" w111 {
              frame False {
              }
              frame True {
                n81 = local write "go straight relative"(FALSE) -> ()
                n82 = local write "key stm"("go straight relative") -> ()
              }
            }
          }
          event "Load sequence": Value Change {
            n83 = event-data() -> ("NewVal"=w114:bool)  [unwired: 1 in, 4 out]
            n84 = case shown="True" w114 {
              frame False {
              }
              frame True {
                n85 = local write "Load sequence"(FALSE) -> ()
                n86 = local write "key stm"("open sequence") -> ()
              }
            }
          }
          event "Normal Betrieb": Value Change {
            n87 = event-data() -> ()  [unwired: 1 in, 5 out]
            n88 = local write "key stm"("initialize" ("key stm")) -> ()
          }
          event "magnetization set": Value Change {
            n89 = event-data() -> ("NewVal"=w118:bool)  [unwired: 1 in, 4 out]
            n90 = case shown="True" w118 {
              frame False {
              }
              frame True {
                n91 = local write "magnetization set"(FALSE) -> ()
                n92 = local write "key stm"("write") -> ()
              }
            }
          }
          event "read": Value Change {
            n93 = event-data() -> ("NewVal"=w121:bool)  [unwired: 1 in, 4 out]
            n94 = case shown="True" w121 {
              frame False {
              }
              frame True {
                n95 = local write "read"(FALSE) -> ()
                n96 = local write "key stm"("read") -> ()
              }
            }
          }
          event "set speed btn": Value Change {
            n97 = event-data() -> ("NewVal"=w124:bool)  [unwired: 1 in, 4 out]
            n98 = case shown="True" w124 {
              frame False {
              }
              frame True {
                n99 = local write "set speed btn"(FALSE) -> ()
                n100 = local write "key stm"("set speed") -> ()
              }
            }
          }
          event "go to reference head": Value Change {
            n101 = event-data() -> ("NewVal"=w127:bool)  [unwired: 1 in, 4 out]
            n102 = case shown="True" w127 {
              frame False {
              }
              frame True {
                n103 = flat-sequence {
                  frame #0 {
                    n104 = local write "temp"("head") -> ()
                  }
                  frame #1 {
                    n105 = local write "key stm"("go to reference") -> ()
                  }
                }
                n106 = local write "go to reference head"(FALSE) -> ()
              }
            }
          }
          event "go to reference kmt": Value Change {
            n107 = event-data() -> ("NewVal"=w131:bool)  [unwired: 1 in, 4 out]
            n108 = case shown="True" w131 {
              frame False {
              }
              frame True {
                n109 = flat-sequence {
                  frame #0 {
                    n110 = local write "temp"("sensor") -> ()
                  }
                  frame #1 {
                    n111 = local write "key stm"("go to reference") -> ()
                  }
                }
                n112 = local write "go to reference kmt"(FALSE) -> ()
              }
            }
          }
          event "save reference head": Value Change {
            n113 = event-data() -> ()  [unwired: 1 in, 5 out]
            n114 = Two Button Dialog(message="Bist Du sicher, dass du den alten Pfad überschreiben möchtest?", 1:"Nein" ("Text für F-Schaltfläche (\"Abbrechen\")"), 2:"Ja" ("Text für T-Schaltfläche (\"OK\")")) -> (T button?=w135:bool)
            n115 = case shown="True" w135 {
              frame False {
              }
              frame True {
                n116 = local write "save reference head"(FALSE) -> ()
                n117 = local read "Reference Write head"() -> (w143:dbl[])
                n118 = Current VI's Path() -> (path=w141:path)
                n119 = Strip Path(path=w141) -> (stripped path=w140:path)  [unwired: 1 out]
                n120 = Build Path(base path=w140, name or relative path="config\\referenz Schreibkopf.txt") -> (appended path=w139:path)
                n121 = call-poly <vilib>:"Write To Spreadsheet File.vi"("1D data"=w143, "file path (dialog if empty)"=w139) -> ()  [unwired: 6 in, 1 out]
              }
            }
          }
          event "go to exchange position": Value Change {
            n122 = event-data() -> ("NewVal"=w145:bool)  [unwired: 1 in, 4 out]
            n123 = case shown="True" w145 {
              frame False {
              }
              frame True {
                n124 = local write "go to exchange position"(FALSE) -> ()
                n125 = local write "key stm"("go to exchange position") -> ()
              }
            }
          }
          event "ED 33 Start": Value Change {
            n126 = event-data() -> ()  [unwired: 1 in, 5 out]
            n127 = local write "key stm 3"("ED33 reset" ("key stm")) -> ()
            n128 = local write "key stm"("ED33 reset" ("key stm")) -> ()
          }
          event "KMT read start": Value Change {
            n129 = event-data() -> ()  [unwired: 1 in, 5 out]
            n130 = local write "key stm 4"("ED33 reset" ("key stm")) -> ()
            n131 = local write "key stm 5"("ED33 reset" ("key stm")) -> ()
            n132 = local write "key stm"("ED33 reset" ("key stm")) -> ()
          }
          event "GAUS read strart 2": Value Change {
            n133 = event-data() -> ()  [unwired: 1 in, 5 out]
            n134 = local write "key stm"("GAUS" ("key stm")) -> ()
          }
          event "open Log": Value Change {
            n135 = event-data() -> ("NewVal"=w154:bool)  [unwired: 1 in, 4 out]
            n136 = case shown="True" w154 {
              frame False {
              }
              frame True {
                n137 = local write "open Log"(FALSE) -> ()
                n138 = local read "sequence path"() -> (w156:path)
                n139 = call-poly <vilib>:"Read From Spreadsheet File.vi"("file path (dialog if empty)"=w156) -> ("all rows"=w155:string[][])  [unwired: 6 in, 4 out]
                n140 = local write "sensor log"(w155) -> ()
              }
            }
          }
          event "save reference kmt": Value Change {
            n141 = event-data() -> ()  [unwired: 1 in, 5 out]
            n142 = Two Button Dialog(message="Bist Du sicher, dass du den alten Pfad überschreiben möchtest?", 1:"Nein" ("Text für F-Schaltfläche (\"Abbrechen\")"), 2:"Ja" ("Text für T-Schaltfläche (\"OK\")")) -> (T button?=w158:bool)
            n143 = case shown="True" w158 {
              frame False {
              }
              frame True {
                n144 = Current VI's Path() -> (path=w163:path)
                n145 = local write "save reference kmt"(FALSE) -> ()
                n146 = Strip Path(path=w163) -> ()  [unwired: 2 out]
                n147 = local read "Referenz KMT"() -> (w166:dbl[])
                n148 = Build Path(name or relative path="config\\referenz KMT.txt") -> (appended path=w162:path)  [unwired: 1 in]
                n149 = call-poly <vilib>:"Write To Spreadsheet File.vi"("1D data"=w166, "file path (dialog if empty)"=w162) -> ()  [unwired: 6 in, 1 out]
              }
            }
          }
          event "set reference head": Value Change {
            n150 = event-data() -> ("NewVal"=w167:bool)  [unwired: 1 in, 4 out]
            n151 = case shown="True" w167 {
              frame False {
              }
              frame True {
                n152 = local write "set reference head"(FALSE) -> ()
                n153 = for {
                  N: 3 -> [_]
                  tunnel: [w171] -> w168 mode=indexing
                  i -> [w172]
                  n154 = local read "current coordinates"() -> (w174:T7)
                  n155 = Cluster To Array(cluster=w174) -> (array=w173:dbl[])
                  n156 = Index Array(array=w173, index=w172) -> (element=w171:dbl)
                }
                n157 = local write "Reference Write head"(w168) -> ()
              }
            }
          }
          event "set reference KMT": Value Change {
            n158 = event-data() -> ("NewVal"=w175:bool)  [unwired: 1 in, 4 out]
            n159 = case shown="True" w175 {
              frame False {
              }
              frame True {
                n160 = local write "set reference KMT"(FALSE) -> ()
                n161 = for {
                  N: 3 -> [_]
                  tunnel: [w179] -> w178 mode=indexing
                  i -> [w180]
                  n162 = local read "current coordinates"() -> (w182:T7)
                  n163 = Cluster To Array(cluster=w182) -> (array=w181:dbl[])
                  n164 = Index Array(array=w181, index=w180) -> (element=w179:dbl)
                }
                n165 = local write "Referenz KMT"(w178) -> ()
              }
            }
          }
          event "clear sensor log": Value Change {
            n166 = event-data() -> ("NewVal"=w183:bool)  [unwired: 1 in, 4 out]
            n167 = case shown="True" w183 {
              frame False {
              }
              frame True {
                n168 = local write "clear sensor log"(FALSE) -> ()
                n169 = local write "sensor log"(string[][] []) -> ()
              }
            }
          }
          event "save log": Value Change {
            n170 = event-data() -> ("NewVal"=w186:bool)  [unwired: 1 in, 4 out]
            n171 = case shown="True" w186 {
              frame False {
              }
              frame True {
                n172 = local write "save log"(TRUE) -> ()
                n173 = local read "sensor log"() -> (w187:string[][])
                n174 = call-poly <vilib>:"Write To Spreadsheet File.vi"("2D data"=w187) -> ()  [unwired: 7 in, 1 out]
              }
            }
          }
          event "clear sequence": Value Change {
            n175 = event-data() -> ("NewVal"=w189:bool)  [unwired: 1 in, 4 out]
            n176 = case shown="True" w189 {
              frame False {
              }
              frame True {
                n177 = local write "clear sequence"(FALSE) -> ()
                n178 = local write "current sequence"(string[] []) -> ()
                n179 = Initialize Array("") -> (w190:string[][])  [unwired: 2 in]
                n180 = local write "sequence"(w190) -> ()
              }
            }
          }
          event "sensor run constant read": Value Change {
            n181 = event-data() -> ("NewVal"=w194:bool)  [unwired: 1 in, 4 out]
            n182 = case shown="True" w194 {
              frame False {
              }
              frame True {
                n183 = local write "sensor run constant read"(FALSE) -> ()
                n184 = local write "key stm"("sensor run constant read") -> ()
              }
            }
          }
          event "Plot": Value Change {
            n185 = event-data() -> ()  [unwired: 1 in, 5 out]
          }
          event "Bereiche  X,Y,Z": Value Change {
            n186 = event-data() -> ()  [unwired: 1 in, 5 out]
            n187 = local write "key stm"("initialize" ("key stm")) -> ()
          }
          event "Standartwiderherstellen Bereiche": Value Change {
            n188 = event-data() -> ()  [unwired: 1 in, 5 out]
            n189 = local write "key stm"("Standart für Bereichsbegrenzug widerherstellen" ("key stm")) -> ()
          }
          event "Set as new standard": Value Change {
            n190 = event-data() -> ()  [unwired: 1 in, 5 out]
            n191 = local write "key stm"("Bereichbegrenzung Werte als neuer Standart setzen" ("key stm")) -> ()
          }
          event "Anwenden": Value Change {
            n192 = event-data() -> ()  [unwired: 1 in, 5 out]
            n193 = local write "key stm"("Bereichsbegrenzung anwenden" ("key stm")) -> ()
          }
          event "Save as text": Value Change {
            n194 = event-data() -> ()  [unwired: 1 in, 5 out]
            n195 = local write "key stm"("Speichern als txt") -> ()
          }
          event "speichern": Value Change {
            n196 = event-data() -> ()  [unwired: 1 in, 5 out]
            n197 = local write "key stm"("Batch Position" ("key stm")) -> ()
          }
          event "Als Standart": Value Change {
            n198 = event-data() -> ()  [unwired: 1 in, 5 out]
            n199 = local write "key stm"("Batch Positionen speichern" ("key stm")) -> ()
          }
          event "bo to batch": Value Change {
            n200 = event-data() -> ()  [unwired: 1 in, 5 out]
            n201 = local write "key stm"("Batch go to position" ("key stm")) -> ()
          }
        }
        n202 = local read "Attached Array"() -> (w36:string[][])
        n203 = global write "Global_Not-Aus.vi" "Not-Aus"("stop program") -> ()
        n204 = Index Array(array=w36, index (col)=0) -> (element=w40:string[])  [unwired: 1 in]
        n205 = Index Array(array=w36, index (col)="Plot") -> (element=w39:string[])  [unwired: 1 in]
        n206 = Decimal String To Number(string=w40) -> (number=w34:i32[])  [unwired: 2 in, 1 out]
        n207 = Decimal String To Number(string=w39) -> (number=w32:i32[])  [unwired: 2 in, 1 out]
        n208 = call "In dynamische Daten konvertieren2"("Array"=w32) -> ("Dynamic Data Type"=w31:dynamicdata)  [unwired: 3 in]
        n209 = call "In dynamische Daten konvertieren"("Array"=w34) -> ("Dynamic Data Type"=w33:dynamicdata)  [unwired: 3 in]
        n210 = call "Build XY Graph"("Y Input"=w31, "X Input"=w33) -> ("XY Graph"=→"XY Graph":cluster{"Y":dbl[], "Y":dbl[]}[])  [unwired: 3 in, 6 out]
        n211 = local read "stop handover"() -> (w43:bool)
      }
      n212 = local read "Port KOSY"() -> (w30:refnum<visa-resource-name>)
      n213 = local read "error IO"() -> (w28:errorcluster)
      n214 = local read "key stm"() -> (w29:string)
      n215 = while {
        shift-right: [w225] -> w27
        shift-left: w28 -> [w210]
        shift-right: [w205] -> _
        shift-left: w29 -> [w209]
        shift-right: [w226] -> _
        shift-left: w30 -> [w206]
        i -> [w207]
        stop <- w227 stop-if-true
        # "sets after each wait-pass key stm\nto auto, so that the next command sequence\ncan be isolated"
        # "processes the command key stm and calls the appropriate routine to the Case structure; if it receives no known keyword, it runs the wait routine"
        # "if sequence active and key stm = auto -> separating the first sequence line\nand forwarding the contents"
        # "if no (sequence array = 0) disable switch \"sequence active?\""
        # "check if sequence-active"
        n216 = local read "sequence"() -> (w211:string[][])
        n217 = local read "key stm"() -> (w217:string)
        n218 = local read "sequence active?"() -> (w216:bool)
        n219 = Array Size(array=w211) -> (size(s)=w223:i32[])
        n220 = Equal?(x=w217, y="auto") -> (x = y?=w213:bool)
        n221 = Index Array(array=w223, index=0) -> (element=w221:i32)
        n222 = Equal?(x=w216, y=TRUE) -> (x = y?=w214:bool)
        n223 = And(x=w213, y=w214) -> (x .and. y?=w212:bool)
        n224 = Equal?(x=w221, y=0) -> (x = y?=w219:bool)
        n225 = case shown="False" w219 {
          frame False {
          }
          frame True {
            n226 = local write "sequence active?"(FALSE) -> ()
          }
        }
        n227 = case shown="True" w212 {
          tunnel: w211 -> [_ w234]
          tunnel: [w228 w229] -> w208
          tunnel: w209 -> [w228 _]
          frame False {
          }
          frame True {
            n228 = Delete From Array(array=w234, index (row)=0) -> (deleted portion=w231:string[], array with subset deleted=w232:string[][])  [unwired: 2 in]
            n229 = local write "sequence"(w232) -> ()
            n230 = local write "current sequence"(w231) -> ()
            n231 = Index Array(array=w231, index=0) -> (element=w229:string)
          }
        }
        n232 = case shown="No Error" w210 {
          selector: w210 -> [w244 w1592]
          tunnel: w206 -> [w247 w1591]
          tunnel: [w246 w1591] -> w226
          tunnel: [w245 w1592] -> w225
          tunnel: [w242 "error"] -> w224
          tunnel: w208 -> [w243 _]
          frame No Error {
            n233 = case shown="\"GAUS\"" w243 {
              selector: w243 -> [_ _ _ _ _ _ _ w388 _ _ _ _ _ _ _ _ _ _ _ _ _ _ _ _ _ _ _ _ _ _ _ _ _ _]
              tunnel: w247 -> [w254 w283 w289 w302 _ w363 w384 w387 w389 w450 w477 w490 w500 w532 w558 w590 w604 w621 _ w723 w735 w737 w825 w852 w896 w1058 w1223 w1401 w1419 w1461 w1503 w1574 w1583 w1587]
              tunnel: w244 -> [w253 w282 w286 w303 w325 w362 w382 w386 w392 w452 w476 w491 w507 w531 w557 w591 w603 w620 w695 w712 w734 w738 w842 w853 w894 w1059 w1226 w1377 w1418 w1460 w1502 w1582 w1586 w1590]
              tunnel: [w252 w283 w289 w302 w322 w363 w383 w387 w394 w449 w464 w489 w498 w525 w543 w590 w604 w621 w694 w723 w724 w737 w825 w847 w895 w1057 w1222 w1401 w1419 w1461 w1503 w1574 w1583 w1587] -> w246
              tunnel: [w251 w282 w286 w303 w324 w362 w381 w386 w397 w451 w465 w488 w506 w524 w556 w591 w603 w620 w695 w712 w733 w738 w842 w850 w888 w1054 w1230 w1377 w1418 w1460 w1502 w1582 w1585 w1589] -> w245
              tunnel: [w250 "wait" "wait" "wait" "wait" "wait" "wait" w388 "wait" "wait" "wait" "wait" "wait" "wait" "wait" "wait" "wait" "wait" "wait" "auto" "wait" "wait" "wait" "wait" "wait" "wait" "wait" "wait" "wait" w1459 "wait" "wait" "wait" "wait"] -> w242
              frame "initialize" {
                n234 = flat-sequence {
                  tunnel: w254 -> [w276]
                  tunnel: w253 -> [w268]
                  tunnel: [w274] -> w249
                  tunnel: [w273] -> w248
                  tunnel: w249 -> [w280]
                  tunnel: w248 -> [w279]
                  tunnel: [w280] -> w252
                  tunnel: [w279] -> w251
                  tunnel: ["wait"] -> w250
                  frame #0 {
                    w271 = TRUE ("read")
                    n235 = local read "Port Netzteil"() -> (w272:refnum<visa-resource-name>)
                    n236 = local read "Batch field memory"() -> (w255:path)
                    n237 = call "Serial_com_powersupply_1.3 (SubVI).vi"("VISA-Referenz (Eingang)"=w272, "read"=w271, "write"=w271) -> ("Initialisiertes Array"=→"Power supply init":string[])  [unwired: 22 in, 2 out]
                    n238 = local read "STM run"() -> (w267:dbl)
                    n239 = call "Werte aus Text lesen.vi"("error in (no error)"=w268, "Dateipfad (Dialog verwenden)"="Choose file spaces") -> ("Cluster"=w266:T15)  [unwired: 7 in, 2 out]
                    n240 = call "Dekoder Batch Speicher.vi"("Batchfeld Speicher"=w255) -> ("P9"=w265:dbl[], "P10"=w256:dbl[], "P1"=w257:dbl[], "P2"=w258:dbl[], "P8"=w264:dbl[], "P3"=w259:dbl[], "P4"=w260:dbl[], "P7"=w263:dbl[], "P6"=w262:dbl[], "P5"=w261:dbl[])  [unwired: 5 in]
                    n241 = local write "p10"(w265) -> ()
                    n242 = local write "p1"(w256) -> ()
                    n243 = local write "p2"(w257) -> ()
                    n244 = local write "p3"(w258) -> ()
                    n245 = local write "p9"(w264) -> ()
                    n246 = local write "p4"(w259) -> ()
                    n247 = local write "p5"(w260) -> ()
                    n248 = local write "p6"(w261) -> ()
                    n249 = local write "p7"(w262) -> ()
                    n250 = local write "p8"(w263) -> ()
                    n251 = local write "Bereiche  X,Y,Z"(w266) -> ()
                    n252 = call "KOSY init4.vi"("error in (no error)"=w268, "Bereiche IF6 X,Y,Z,U,C,A,B\n(X:0-310,Y:0-275,Z:0-108,U:0,C:0,A:0,B:0)"=w266, "Numerisch"=w267, "VISA-Referenz (Eingang)"=w276) -> ("Fehler (Ausgang)"=w273:errorcluster, "Coordinates IF6"=w275:T16, "VISA-Referenz (Ausgang)"=w274:refnum<visa-resource-name>)  [unwired: 4 in, 1 out]
                    n253 = local write "current coordinates"(w275) -> ()
                  }
                  frame #1 {
                    n254 = local write "key stm"("Set Ed33 initial position") -> ()
                  }
                }
              }
              frame "Restore Default for range restriction" {
                n255 = flat-sequence {
                  frame #0 {
                    n256 = local write "Bereiche  X,Y,Z"("Standard memory") -> ()
                  }
                  frame #1 {
                    n257 = local write "key stm"("initialize" ("key stm")) -> ()
                  }
                }
              }
              frame "Set range limit values as the new standard" {
                n258 = flat-sequence {
                  tunnel: [w290] -> w287
                  tunnel: w287 -> [w292]
                  frame #0 {
                    n259 = local read "Bereiche  X,Y,Z"() -> (w290:T2)
                    n260 = local write "Standard memory"(w290) -> ()
                  }
                  frame #1 {
                    n261 = local read "Choose file spaces"() -> (w291:path)
                    n262 = call "Werte in Text schreiben.vi"("Path"=w291, "Bereiche  X,Y,Z"=w292) -> ()  [unwired: 10 in]
                  }
                  frame #2 {
                    n263 = local write "key stm"("Restore Default for range restriction" ("key stm")) -> ()
                  }
                }
              }
              frame "Batch Position" {
                n264 = local write "key stm"("auto" ("key stm")) -> ()
                n265 = local read "current coordinates"() -> (w300:T7)
                n266 = Unbundle(w300) -> ("steps x"=w299:dbl, "steps y"=w298:dbl, "steps z"=w297:dbl)  [unwired: 4 out]
                n267 = Build Array(w299, w298, w297) -> (w296:dbl[])
                n268 = case shown="False" "speichern" {
                  tunnel: w296 -> [w304 _]
                  frame False {
                    n269 = case shown="\"Position 2\"" "Enum" {
                      tunnel: w304 -> [w306 w307 w308 w309 w310 w311 w312 w313 w314 w315]
                      frame "Position 1", Default {
                        n270 = local write "p1"(w306) -> ()
                      }
                      frame "Position 2" {
                        n271 = local write "p2"(w307) -> ()
                      }
                      frame "Position 3" {
                        n272 = local write "p3"(w308) -> ()
                      }
                      frame "Position 4" {
                        n273 = local write "p4"(w309) -> ()
                      }
                      frame "Position 5" {
                        n274 = local write "p5"(w310) -> ()
                      }
                      frame "Position 6" {
                        n275 = local write "p6"(w311) -> ()
                      }
                      frame "Position 7" {
                        n276 = local write "p7"(w312) -> ()
                      }
                      frame "Position 8" {
                        n277 = local write "p8"(w313) -> ()
                      }
                      frame "Position 9" {
                        n278 = local write "p9"(w314) -> ()
                      }
                      frame "Position 10" {
                        n279 = local write "p10"(w315) -> ()
                      }
                    }
                  }
                  frame True {
                  }
                }
              }
              frame "Batch go to position" {
                n280 = local read "current sequence"() -> (w321:string[])
                n281 = local read "sequence active?"() -> (w318:bool)
                n282 = Or(x="bo to batch", y=w318) -> (x .or. y?=w317:bool)
                n283 = Index Array(array=w321, index=1 ("Index")) -> (element=w319:string)
                n284 = case shown="\"p10\"" w319 {
                  frame "False", Default {
                  }
                  frame "p1" {
                    n285 = local write "Enum 2"(T9."p1" ("Enum 2")) -> ()
                  }
                  frame "p2" {
                    n286 = local write "Enum 2"(T9."p2" ("Enum 2")) -> ()
                  }
                  frame "p3" {
                    n287 = local write "Enum 2"(T9."p3" ("Enum 2")) -> ()
                  }
                  frame "p4" {
                    n288 = local write "Enum 2"(T9."p4" ("Enum 2")) -> ()
                  }
                  frame "p5" {
                    n289 = local write "Enum 2"(T9."p5" ("Enum 2")) -> ()
                  }
                  frame "p6" {
                    n290 = local write "Enum 2"(T9."p6" ("Enum 2")) -> ()
                  }
                  frame "p7" {
                    n291 = local write "Enum 2"(T9."p7" ("Enum 2")) -> ()
                  }
                  frame "p8" {
                    n292 = local write "Enum 2"(T9."p8" ("Enum 2")) -> ()
                  }
                  frame "p9" {
                    n293 = local write "Enum 2"(T9."p9" ("Enum 2")) -> ()
                  }
                  frame "p10" {
                    n294 = local write "Enum 2"(T9."p10" ("Enum 2")) -> ()
                  }
                }
                n295 = case shown="True" w317 {
                  tunnel: w325 -> [w336 w342]
                  tunnel: [w336 w341] -> w324
                  tunnel: [w337 w338] -> w322
                  frame False {
                    n296 = local read "Port KOSY"() -> (w337:refnum<visa-resource-name>)
                  }
                  frame True {
                    n297 = case shown="\"p1\", Default" "Enum 2" {
                      tunnel: [w350 w351 w352 w353 w354 w355 w356 w357 w358 w359] -> w340
                      frame "p1", Default {
                        n298 = local read "p1"() -> (w350:dbl[])
                      }
                      frame "p3" {
                        n299 = local read "p3"() -> (w351:dbl[])
                      }
                      frame "p4" {
                        n300 = local read "p4"() -> (w352:dbl[])
                      }
                      frame "p5" {
                        n301 = local read "p5"() -> (w353:dbl[])
                      }
                      frame "p6" {
                        n302 = local read "p6"() -> (w354:dbl[])
                      }
                      frame "p7" {
                        n303 = local read "p7"() -> (w355:dbl[])
                      }
                      frame "p8" {
                        n304 = local read "p8"() -> (w356:dbl[])
                      }
                      frame "p9" {
                        n305 = local read "p9"() -> (w357:dbl[])
                      }
                      frame "p10" {
                        n306 = local read "p10"() -> (w358:dbl[])
                      }
                      frame "p2" {
                        n307 = local read "p2"() -> (w359:dbl[])
                      }
                    }
                    n308 = local read "speed"() -> (w346:dbl)
                    n309 = local read "current coordinates"() -> (w344:T7)
                    n310 = local read "Port KOSY"() -> (w349:refnum<visa-resource-name>)
                    n311 = Bundle(1, "speed"=w346, 1) -> (w345:cluster{i32, "speed":dbl, i32})  [unwired: 1 in]
                    n312 = call <userlib>:"SubVI_Punkt_anfahren_IF5_IF6.vi"("Angehängtes Array"=w340, "error in"=w342, "Koordinaten in IF6"=w344, "Geschwindigkeiten"=w345, "VISA resource name in"=w349) -> ("error out"=w341:errorcluster, "Koordinaten out IF6"=w343:T16, "VISA resource name in 2"=w338:refnum<visa-resource-name>)  [unwired: 1 in]
                    n313 = local write "current coordinates"(w343) -> ()
                  }
                }
              }
              frame "Save batch positions" {
                n314 = case shown="True" "Als Standart" {
                  frame False {
                  }
                  frame True {
                    n315 = local read "p10"() -> (w370:dbl[])
                    n316 = local read "p1"() -> (w366:dbl[])
                    n317 = local read "p2"() -> (w365:dbl[])
                    n318 = local read "p3"() -> (w364:dbl[])
                    n319 = local read "p3"() -> (w377:dbl[])
                    n320 = local read "p4"() -> (w376:dbl[])
                    n321 = local read "p5"() -> (w375:dbl[])
                    n322 = local read "p6"() -> (w374:dbl[])
                    n323 = local read "p7"() -> (w373:dbl[])
                    n324 = local read "p8"() -> (w372:dbl[])
                    n325 = local read "p9"() -> (w371:dbl[])
                    n326 = Build Array(w366, w365, w364, w377, w376, w375, w374, w373, w372, w371, w370) -> (w369:dbl[][])
                    n327 = call-poly <vilib>:"Write To Spreadsheet File.vi"("format (%.3f)"="%.6f", "2D data"=w369, "file path (dialog if empty)"="Batch field memory") -> ()  [unwired: 5 in, 1 out]
                  }
                }
              }
              frame "Apply range limitation" {
                n328 = local read "Bereiche  X,Y,Z"() -> (w380:T2)
                n329 = call "SubVI_Setze_Bereiche_IF5_IF6.vi"("VISA resource name in"=w384, "Bereiche IF6 X,Y,Z,U,C,A,B\n(X:0-310,Y:0-275,Z:0-108,U:0,C:0,A:0,B:0)"=w380, "IF5=F/IF6=T\n(IF6=T) in"=TRUE ("IF5=F/IF6=T\n(IF6=T) in"), "error in"=w382) -> ("VISA resource name out"=w383:refnum<visa-resource-name>, "error out"=w381:errorcluster)  [unwired: 8 in, 2 out]
              }
              frame "wait", Default {
                # "standard process, wait 50ms"
                n330 = Wait (ms)(milliseconds to wait=50) -> ()  [unwired: 1 out]
              }
              frame "manual control" {
                # "Routine for manual control of the stage movement.\nGets the parameters of the movement from the event \"button\"\nfrom the event structure"
                n331 = flat-sequence {
                  tunnel: w389 -> [w411]
                  tunnel: w392 -> [w410]
                  tunnel: [w411] -> w409
                  tunnel: [w410] -> w408
                  tunnel: w409 -> [w414]
                  tunnel: w408 -> [w413]
                  tunnel: [w418] -> w407
                  tunnel: [w417] -> w406
                  tunnel: [w416] -> w405
                  tunnel: [w415] -> w404
                  tunnel: [w414] -> w403
                  tunnel: [w413] -> w402
                  tunnel: w407 -> [w428]
                  tunnel: w406 -> [w427]
                  tunnel: w405 -> [w420]
                  tunnel: w404 -> [w426]
                  tunnel: w403 -> [w425]
                  tunnel: w402 -> [w421]
                  tunnel: [w422] -> w401
                  tunnel: [w424] -> w400
                  tunnel: [w423] -> w395
                  tunnel: w401 -> [w430]
                  tunnel: w400 -> [w432]
                  tunnel: [w430] -> w398
                  tunnel: [w429] -> w396
                  tunnel: w395 -> [w429]
                  tunnel: cluster{u16, u16, dbl, bool} {36, 1, 0.0, TRUE} -> [w435]
                  tunnel: w398 -> [w434]
                  tunnel: w396 -> [w433]
                  tunnel: [w434] -> w391
                  tunnel: [w433] -> w390
                  tunnel: [w438] -> w394
                  tunnel: [w436] -> w397
                  tunnel: w391 -> [w436]
                  tunnel: w390 -> [w438]
                  frame #0 {
                    n332 = local write "moving"(TRUE) -> ()
                  }
                  frame #1 {
                    n333 = local read "movement"() -> (w419:T10)
                    n334 = Unbundle(w419) -> ("Achsen-Wahl (X)"=w418:u8, "Richtung (vEw)"=w417:u8, "Geschwindigkeit\nin mm/s (5)[0,025-20]"=w416:sgl, "IV6"=w415:bool)
                  }
                  frame #2 {
                    n335 = call <userlib>:"SubVI_Einzelschritte_IF5_IF6.vi"("VISA resource name in"=w425, "Achsen-Wahl (X)"=w428, "Geschwindigkeit\nin mm/s (5)[0,025-20]"=w420, "IF5=F/IF6=T\n(IF6=T) in"=w426, "error in"=w421, "Richtung (vEw)"=w427) -> ("VISA resource name out"=w423:refnum<visa-resource-name>, "Koordinaten IF6"=w424:T16, "error out"=w422:errorcluster)  [unwired: 3 in, 4 out]
                  }
                  frame #3 {
                    n336 = local write "current coordinates"(w432) -> ()
                    n337 = Wait (ms)(milliseconds to wait=100) -> ()  [unwired: 1 out]
                  }
                  frame #4 {
                    n338 = local write "movement"(w435) -> ()
                  }
                  frame #5 {
                    n339 = local write "key stm"("Aktuelle Position ED33" ("key stm")) -> ()
                  }
                }
              }
              frame "go to coordinates" {
                # "Drive to the coordinates from sequence or array of manual\nControl. First moves the Z axis to zero before the movement\ntakes place in the x-and y-direction"
                n340 = local read "sequence active?"() -> (w443:bool)
                n341 = Equal?(x=w443, y=TRUE) -> (x = y?=w445:bool)
                n342 = case shown="True" w445 {
                  tunnel: [w454 w455] -> w453
                  frame False {
                    n343 = local read "coordinates"() -> (w454:dbl[])
                  }
                  frame True {
                    n344 = for {
                      N: 3 -> [_]
                      tunnel: [w457] -> w455 mode=indexing
                      i -> [w460]
                      n345 = local read "current sequence"() -> (w462:string[])
                      n346 = Add(x=1, y=w460) -> (x+y=w459:i32)
                      n347 = Index Array(array=w462, index=w459) -> (element=w458:string)
                      n348 = Fract/Exp String To Number(string=w458) -> (number=w457:dbl)  [unwired: 3 in, 1 out]
                    }
                  }
                }
                n349 = local read "current coordinates"() -> (w448:T7)
                n350 = local read "speed"() -> (w442:dbl)
                n351 = Bundle(1, "speed"=w442, 1) -> (w439:cluster{i32, "speed":dbl, i32})  [unwired: 1 in]
                n352 = call <userlib>:"SubVI_Multi_linear_interpolation_IF5_IF6.vi"("new position"=w453, "error in"=w452, "coordinates in IF6"=w448, "speed"=w439, "VISA resource name in"=w450) -> ("error out"=w451:errorcluster, "coordinates out IF6"=w447:T16, "VISA resource name in 2"=w449:refnum<visa-resource-name>)  [unwired: 1 in]
                n353 = local write "current coordinates"(w447) -> ()
              }
              frame "go to exchange position" {
                # "moves to a position in which the replacement of the magnetic tapes is facilitated"
                n354 = local read "current coordinates"() -> (w471:T7)
                n355 = Build Array(0.0 ("Element"), 250.0 ("Element"), 0.0 ("Element")) -> (w472:dbl[])
                n356 = Bundle("Element"=1.0, "Element"=15.0, "Element"=1.0) -> (w467:T17)  [unwired: 1 in]
                n357 = call <userlib>:"SubVI_Multi_linear_interpolation_IF5_IF6.vi"("new position"=w472, "error in"=w476, "coordinates in IF6"=w471, "speed"=w467, "VISA resource name in"=w477) -> ("error out"=w465:errorcluster, "coordinates out IF6"=w466:T16, "VISA resource name in 2"=w464:refnum<visa-resource-name>)  [unwired: 1 in]
                n358 = local write "current coordinates"(w466) -> ()
              }
              frame "go to reference" {
                # "moves to the stored reference position for write or read operation"
                n359 = local read "sequence active?"() -> (w478:bool)
                n360 = case shown="False" w478 {
                  tunnel: [w492 w493] -> w480
                  frame False {
                    n361 = local read "temp"() -> (w492:string)
                  }
                  frame True {
                    n362 = local read "current sequence"() -> (w495:string[])
                    n363 = Index Array(array=w495, index=1) -> (element=w493:string)
                  }
                }
                n364 = case shown="\"head\", Default" w480 {
                  tunnel: [w496 w497] -> w487
                  frame "head", Default {
                    n365 = local read "Reference Write head"() -> (w496:dbl[])
                  }
                  frame "sensor" {
                    n366 = local read "Referenz KMT"() -> (w497:dbl[])
                  }
                }
                n367 = local read "current coordinates"() -> (w482:T7)
                n368 = local read "speed"() -> (w484:dbl)
                n369 = Bundle(1, "speed"=w484, 1) -> (w483:cluster{i32, "speed":dbl, i32})  [unwired: 1 in]
                n370 = call <userlib>:"SubVI_Multi_linear_interpolation_IF5_IF6.vi"("new position"=w487, "error in"=w491, "coordinates in IF6"=w482, "speed"=w483, "VISA resource name in"=w490) -> ("error out"=w488:errorcluster, "coordinates out IF6"=w481:T16, "VISA resource name in 2"=w489:refnum<visa-resource-name>)  [unwired: 1 in]
                n371 = local write "current coordinates"(w481) -> ()
              }
              frame "go straight to coordinates" {
                # "Direct drive to the coordinates from sequence or array of manual\nControl. No movement of the Z-axis at zero."
                n372 = local read "sequence active?"() -> (w512:bool)
                n373 = Equal?(x=w512, y=TRUE) -> (x = y?=w510:bool)
                n374 = case shown="True" w510 {
                  tunnel: [w513 w514] -> w509
                  frame False {
                    n375 = local read "coordinates"() -> (w513:dbl[])
                  }
                  frame True {
                    n376 = for {
                      N: 3 -> [_]
                      tunnel: [w516] -> w514 mode=indexing
                      i -> [w520]
                      n377 = local read "current sequence"() -> (w521:string[])
                      n378 = Add(x=1, y=w520) -> (x+y=w518:i32)
                      n379 = Index Array(array=w521, index=w518) -> (element=w517:string)
                      n380 = Fract/Exp String To Number(string=w517) -> (number=w516:dbl)  [unwired: 3 in, 1 out]
                    }
                  }
                }
                n381 = local read "speed"() -> (w501:dbl)
                n382 = local read "current coordinates"() -> (w508:T7)
                n383 = Bundle(1, "speed"=w501, 1) -> (w499:cluster{i32, "speed":dbl, i32})  [unwired: 1 in]
                n384 = call <userlib>:"SubVI_Multi_linear_interpolation_IF5_IF6.vi"("new position"=w509, "error in"=w507, "coordinates in IF6"=w508, "speed"=w499, "VISA resource name in"=w500) -> ("error out"=w506:errorcluster, "coordinates out IF6"=w505:T16, "VISA resource name in 2"=w498:refnum<visa-resource-name>)  [unwired: 1 in]
                n385 = local write "current coordinates"(w505) -> ()
              }
              frame "go relative" {
                w530 = cluster{dbl, dbl, dbl, dbl, dbl, dbl, dbl} {0.0, 0.0, 0.0, 0.0, 0.0, 0.0, 0.0}  # zero coordinates
                # "Motion by a specified value, based on the current\nPosition. Works strangely not properly"
                n386 = local read "sequence active?"() -> (w534:bool)
                n387 = case shown="True" w534 {
                  tunnel: [w535 w536] -> w533
                  frame False {
                    n388 = local read "coordinates"() -> (w535:dbl[])
                  }
                  frame True {
                    n389 = for {
                      N: 3 -> [_]
                      tunnel: [w538] -> w536 mode=indexing
                      i -> [w541]
                      n390 = local read "current sequence"() -> (w542:string[])
                      n391 = Increment(x=w541) -> (x+1=w540:i32)
                      n392 = Index Array(array=w542, index=w540) -> (element=w539:string)
                      n393 = Fract/Exp String To Number(string=w539) -> (number=w538:dbl)  [unwired: 3 in, 1 out]
                    }
                  }
                }
                n394 = local read "speed"() -> (w527:dbl)
                n395 = Bundle(0, "speed"=w527, 0) -> (w526:cluster{i32, "speed":dbl, i32})  [unwired: 1 in]
                n396 = call <userlib>:"SubVI_Multi_linear_interpolation_IF5_IF6.vi"("new position"=w533, "error in"=w531, "coordinates in IF6"=w530, "speed"=w526, "VISA resource name in"=w532) -> ("error out"=w524:errorcluster, "coordinates out IF6"=w523:T16, "VISA resource name in 2"=w525:refnum<visa-resource-name>)  [unwired: 1 in]
                n397 = local write "current coordinates"(w523) -> ()
              }
              frame "go straight relative" {
                # "direct motion by a specified value, based on the current\nposition"
                n398 = flat-sequence {
                  tunnel: [w568] -> w544
                  tunnel: [w567] -> w549
                  tunnel: [w566] -> w548
                  tunnel: [w559] -> w545
                  frame #0 {
                    n399 = local read "sequence active?"() -> (w573:bool)
                    n400 = Equal?(x=w573, y=TRUE) -> (x = y?=w571:bool)
                    n401 = case shown="True" w571 {
                      tunnel: [w580 w581] -> w570
                      frame False {
                        n402 = local read "coordinates"() -> (w580:dbl[])
                      }
                      frame True {
                        n403 = for {
                          N: 7 -> [_]
                          tunnel: [w583] -> w581 mode=indexing
                          i -> [w586]
                          n404 = local read "current sequence"() -> (w588:string[])
                          n405 = Add(x=1, y=w586) -> (x+y=w585:i32)
                          n406 = Index Array(array=w588, index=w585) -> (element=w584:string)
                          n407 = Fract/Exp String To Number(string=w584) -> (number=w583:dbl)  [unwired: 3 in, 1 out]
                        }
                      }
                    }
                    n408 = Array To Cluster(array=w570) -> (cluster=w569:T18)
                    n409 = Unbundle(w569) -> ("coordinates[0]"=w568:dbl, "coordinates[1]"=w567:dbl, "coordinates[2]"=w566:dbl, "coordinates[3]"=w565:dbl, "coordinates[4]"=w564:dbl, "coordinates[5]"=w563:dbl)  [unwired: 3 out]
                    n410 = case shown="0, Default" w565 {
                      tunnel: [T13."zum Endschalter hin" T14."zum Endschalter hin"] -> w562
                      frame 0, Default {
                      }
                      frame 1 {
                      }
                    }
                    n411 = case shown="1" w564 {
                      tunnel: [T13."vom Endschalter weg" T13."zum Endschalter hin"] -> w561
                      frame 0, Default {
                      }
                      frame 1 {
                      }
                    }
                    n412 = case shown="1" w563 {
                      tunnel: [T13."vom Endschalter weg" T13."zum Endschalter hin"] -> w560
                      frame 0, Default {
                      }
                      frame 1 {
                      }
                    }
                    n413 = Bundle(w562, w561, w560) -> (w559:T19)  [unwired: 1 in]
                  }
                }
                n414 = local read "speed"() -> (w551:dbl)
                n415 = Bundle("coordinates[0]"=w544, "coordinates[1]"=w549, "coordinates[2]"=w548) -> (w546:T20)  [unwired: 1 in]
                n416 = Bundle(8, "speed"=w551, 0) -> (w552:cluster{i32, "speed":dbl, i32})  [unwired: 1 in]
                n417 = call <userlib>:"SubVI_Geradeninterpolation_3_Achs_IF5_IF6.vi"("VISA resource name in"=w558, "Geschwindigkeiten"=w552, "IF5=F/IF6=T\n(IF6=T) in"=TRUE ("IF5=F/IF6=T\n(IF6=T) in"), "Abstände"=w546, "error in"=w557, "Richtungen"=w545) -> ("VISA resource name out"=w543:refnum<visa-resource-name>, "Koordinaten IF6"=w550:T16, "error out"=w556:errorcluster)  [unwired: 4 in, 3 out]
                n418 = local write "current coordinates"(w550) -> ()
              }
              frame "set speed" {
                # "sets the variable \"speed\" to the specified value"
                n419 = local read "sequence active?"() -> (w595:bool)
                n420 = Equal?(x=w595, y=TRUE) -> (x = y?=w593:bool)
                n421 = case shown="True" w593 {
                  tunnel: [w596 w597] -> w592
                  frame False {
                    n422 = local read "set speed"() -> (w596:dbl)
                  }
                  frame True {
                    n423 = local read "current sequence"() -> (w600:string[])
                    n424 = Index Array(array=w600, index=1) -> (element=w598:string)
                    n425 = Fract/Exp String To Number(string=w598) -> (number=w597:dbl)  [unwired: 3 in, 1 out]
                  }
                }
                n426 = local write "speed"(w592) -> ()
              }
              frame "set powersuply" {
                n427 = local read "sequence active?"() -> (w601:bool)
                n428 = case shown="True" w601 {
                  frame False {
                  }
                  frame True {
                    n429 = local read "current sequence"() -> (w608:string[])
                    n430 = Index Array(array=w608, index=1 ("Index")) -> (element=w607:string)
                    n431 = local read "Port Netzteil"() -> (w610:refnum<visa-resource-name>)
                    n432 = Concatenate Strings(w607, "\r") -> (w605:string)
                    n433 = call "Serial_com_powersupply für Funktion.vi"("VISA resource name"=w610, "write"=TRUE, "string to write"=w605) -> ()  [unwired: 6 in, 2 out]
                  }
                }
              }
              frame "write" {
                # "Communicating with the relay circuit of the solenoid. Presented the parameter \"O\", \"P\" or \"N\" to the controller further\nand controls the direction of current flow within the coil and hence the direction of magnetization"
                n434 = local read "sequence active?"() -> (w625:bool)
                n435 = Equal?(x=w625, y=TRUE) -> (x = y?=w612:bool)
                n436 = case shown="True" w612 {
                  tunnel: [w628 w661] -> w623
                  frame False {
                    n437 = local read "Second head On/Off"() -> (w626:bool)
                    n438 = local read "magnetization"() -> (w629:u16)
                    n439 = local read "Port Netzteil"() -> (w627:refnum<visa-resource-name>)
                    n440 = case shown="0, Default" w629 {
                      tunnel: ["O" w635 w648] -> w628
                      tunnel: w627 -> [_ w634 w646]
                      tunnel: w626 -> [_ w633 w647]
                      frame 0, Default {
                        # "Netzteil sperren aus"
                        n441 = call "Serial_com_powersupply_on off (SubVI).vi"("VISA-Referenz (Eingang)"="Port Netzteil", "string to write"="GOUT 0\r") -> ()  [unwired: 25 in, 1 out]
                      }
                      frame 1 {
                        n442 = case shown="False" w633 {
                          tunnel: ["qw" "qwer"] -> w635
                          tunnel: w634 -> [w636 w640]
                          frame False {
                            n443 = call "Serial_com_powersupply_1.0 zweiten Kopf an aus (SubVI).vi"("VISA-Referenz (Eingang)"=w636, "string to write 3"="OUT 1\r", "string to write"="ADR 00\r") -> ()  [unwired: 22 in, 3 out]
                          }
                          frame True {
                            n444 = call "Serial_com_powersupply_1.1 zweiten Kopf an aus (SubVI).vi"("VISA-Referenz (Eingang)"=w640, "Element 2"="OUT 1\r", "string to write 3"="OUT 1\r", "string to write"="ADR 00\r", "Element"="ADR 01\r") -> ()  [unwired: 20 in, 3 out]
                          }
                        }
                      }
                      frame 2 {
                        n445 = case shown="False" w647 {
                          tunnel: ["12" "1234"] -> w648
                          tunnel: w646 -> [w651 w657]
                          frame False {
                            n446 = call "Serial_com_powersupply_1.0 zweiten Kopf an aus (SubVI).vi"("VISA-Referenz (Eingang)"=w651, "string to write 3"="OUT 1\r", "string to write"="ADR 00\r") -> ()  [unwired: 22 in, 3 out]
                          }
                          frame True {
                            n447 = call "Serial_com_powersupply_1.1 zweiten Kopf an aus (SubVI).vi"("VISA-Referenz (Eingang)"=w657, "Element 2"="OUT 1\r", "string to write 3"="OUT 1\r", "string to write"="ADR 00\r", "Element"="ADR 01\r") -> ()  [unwired: 20 in, 3 out]
                          }
                        }
                      }
                    }
                  }
                  frame True {
                    n448 = local read "Second head On/Off"() -> (w660:bool)
                    n449 = local read "current sequence"() -> (w664:string[])
                    n450 = local read "Port Netzteil"() -> (w659:refnum<visa-resource-name>)
                    n451 = Index Array(array=w664, index=1) -> (element=w662:string)
                    n452 = case shown="\"N\"" w662 {
                      tunnel: [w667 w680 "O"] -> w661
                      tunnel: w660 -> [w665 w678 _]
                      tunnel: w659 -> [w666 w679 w691]
                      frame "P" {
                        n453 = case shown="False" w665 {
                          tunnel: ["1234" "1234"] -> w667
                          tunnel: w666 -> [w668 w672]
                          frame False {
                            n454 = call "Serial_com_powersupply_1.0 zweiten Kopf an aus (SubVI).vi"("VISA-Referenz (Eingang)"=w668, "string to write 3"="OUT 1\r", "string to write"="ADR 00\r") -> ()  [unwired: 22 in, 3 out]
                          }
                          frame True {
                            n455 = call "Serial_com_powersupply_1.1 zweiten Kopf an aus (SubVI).vi"("VISA-Referenz (Eingang)"=w672, "Element 2"="OUT 1\r", "string to write 3"="OUT 1\r", "string to write"="ADR 00\r", "Element"="ADR 01\r") -> ()  [unwired: 20 in, 3 out]
                          }
                        }
                      }
                      frame "N" {
                        n456 = case shown="False" w678 {
                          tunnel: ["qwer" "qwer"] -> w680
                          tunnel: w679 -> [w683 w685]
                          frame False {
                            n457 = call "Serial_com_powersupply_1.0 zweiten Kopf an aus (SubVI).vi"("VISA-Referenz (Eingang)"=w683, "string to write 3"="OUT 1\r", "string to write"="ADR 00\r") -> ()  [unwired: 22 in, 3 out]
                          }
                          frame True {
                            n458 = call "Serial_com_powersupply_1.1 zweiten Kopf an aus (SubVI).vi"("VISA-Referenz (Eingang)"=w685, "Element 2"="OUT 1\r", "string to write 3"="OUT 1\r", "string to write"="ADR 00\r", "Element"="ADR 01\r") -> ()  [unwired: 20 in, 3 out]
                          }
                        }
                      }
                      frame "O", Default {
                        n459 = call "Serial_com_powersupply_on off (SubVI).vi"("VISA-Referenz (Eingang)"=w691, "string to write"="GOUT 0\r") -> ()  [unwired: 25 in, 1 out]
                      }
                    }
                  }
                }
                n460 = local read "Port Write head"() -> (w618:refnum<visa-resource-name>)
                n461 = call-poly "VISA Configure Serial Port"("VISA resource name"=w618, "baud rate (9600)"=9600) -> ("VISA resource name out"=w616:refnum<visa-resource-name>, "error out"=w617:errorcluster)  [unwired: 12 in]
                n462 = call "Serielle Schnittstelle 1.vi"("Fehler (Eingang)"=w617, "Write"=w623, "VISA-Ressourcenname"=w616) -> ("Fehler (Ausgang)"=w614:errorcluster, "Read"=w622:string, "VISA-Ressourcenname 2"=w615:refnum<visa-resource-name>)  [unwired: 5 in]
                n463 = VISA Close(VISA resource name=w615, error in (no error)=w614) -> ()  [unwired: 1 out]
                n464 = local write "Write head Output"(w622) -> ()
              }
              frame "Second head" {
                n465 = local read "sequence active?"() -> (w699:bool)
                n466 = case shown="True" w699 {
                  tunnel: [dbl[] [] w702] -> w698
                  frame False {
                  }
                  frame True {
                    n467 = for {
                      N: 2 -> [_]
                      tunnel: [w707] -> w702 mode=indexing
                      i -> [w704]
                      n468 = local read "current sequence"() -> (w709:string[])
                      n469 = Add(x=1.0, y=w704) -> (x+y=w706:dbl)
                      n470 = Index Array(array=w709, index=w706) -> (element=w708:string)
                      n471 = Fract/Exp String To Number(string=w708) -> (number=w707:dbl)  [unwired: 3 in, 1 out]
                    }
                  }
                }
                n472 = Array To Cluster(array=w698) -> (cluster=w697:T21)
                n473 = Unbundle(w697) -> ("[0]"=w696:dbl)  [unwired: 8 out]
                n474 = case shown="1" w696 {
                  frame 0, Default {
                    n475 = local write "Second head On/Off"(FALSE ("Zweiter Kopf AN/AUS")) -> ()
                  }
                  frame 1 {
                    n476 = local write "Second head On/Off"(TRUE ("Zweiter Kopf AN/AUS")) -> ()
                  }
                }
                n477 = local read "Port KOSY"() -> (w694:refnum<visa-resource-name>)
              }
              frame "ED33 Schreiben" {
                n478 = local read "current sequence"() -> (w721:string[])
                n479 = local write "key stm"("Current position Ed33" ("key stm")) -> ()
                n480 = Index Array(array=w721, index=1 ("Index")) -> (element=w719:string)
                n481 = local read "Port ED33"() -> (w722:refnum<visa-resource-name>)
                n482 = Decimal String To Number(string=w719, default (0L)=0.0 ("Standard (0 I32)")) -> (number=w718:dbl)  [unwired: 1 in, 1 out]
                n483 = local read "speed"() -> (w714:dbl)
                n484 = call "ED33_1.0 Schreiben (SubVI).vi"("VISA-Referenz (Eingang)"=w722, "error in"=w712, "speed 2"=w714, "Pollänge"=w718) -> ("Koordinaten IF6"=w716:T16)  [unwired: 17 in, 6 out]
                n485 = local write "current coordinates"(w716) -> ()
              }
              frame "go straight to reference" {
                n486 = local read "Reference Write head"() -> (w732:dbl[])
                n487 = local read "current coordinates"() -> (w727:T7)
                n488 = local read "speed"() -> (w729:dbl)
                n489 = Bundle(1, "speed"=w729, 1) -> (w728:cluster{i32, "speed":dbl, i32})  [unwired: 1 in]
                n490 = call <userlib>:"SubVI_Multi_linear_interpolation_IF5_IF6.vi"("new position"=w732, "error in"=w734, "coordinates in IF6"=w727, "speed"=w728, "VISA resource name in"=w735) -> ("error out"=w733:errorcluster, "coordinates out IF6"=w726:T16, "VISA resource name in 2"=w724:refnum<visa-resource-name>)  [unwired: 1 in]
                n491 = local write "current coordinates"(w726) -> ()
              }
              frame "open sequence" {
                n492 = flat-sequence {
                  frame #0 {
                    n493 = local write "path Selection"(T1."0" ("Pfadauswahl")) -> ()
                  }
                  frame #1 {
                    n494 = for {
                      N: 20 -> [_]
                      n495 = case shown="\"0\", Default" "path Selection" {
                        tunnel: ["Pfad 20" "Pfad 1" "Pfad 2" "Pfad2" "Pfad 4" "Pfad 5" "Pfad 6" "Pfad 7" "Pfad 8" "Pfad 9" "Pfad 10" "Pfad 11" "Pfad 12" "Pfad 13" "Pfad 14" "Pfad 15" "Pfad 16" "Pfad 17" "Pfad 18" "Pfad 19" "Pfad 0"] -> w745
                        tunnel: ["Boolesch1 24" "Boolesch1" "Boolesch1 25" "Boolesch1 2" "Boolesch1 3" "Boolesch1" "Boolesch1" "Boolesch1 17" "Boolesch1 16" "Boolesch1 15" "Boolesch1 14" "Boolesch1 13" "Boolesch1 12" "Boolesch1 11" "Boolesch1 18" "Boolesch1 19" "Boolesch1 20" "Boolesch1 21" "Boolesch1 22" "Boolesch1 23" "Boolesch1"] -> w744
                        tunnel: [T1."1" ("Pfadauswahl 2") T1."2" ("Pfadauswahl 2") T1."3" ("Pfadauswahl 2") T1."4" ("Pfadauswahl 2") T1."5" ("Pfadauswahl 2") T1."6" ("Pfadauswahl 2") T1."7" ("Pfadauswahl 2") T1."8" ("Pfadauswahl 2") T1."9" ("Pfadauswahl 2") T1."10" ("Pfadauswahl 2") T1."11" ("Pfadauswahl 2") T1."12" ("Pfadauswahl 2") T1."13" ("Pfadauswahl 2") T1."14" ("Pfadauswahl 2") T1."15" ("Pfadauswahl 2") T1."16" ("Pfadauswahl 2") T1."17" ("Pfadauswahl 2") T1."18" ("Pfadauswahl 2") T1."19" ("Pfadauswahl 2") T1."20" ("Pfadauswahl 2") T1."0" ("Pfadauswahl 2")] -> w742
                        frame "0", Default {
                        }
                        frame "1" {
                        }
                        frame "2" {
                        }
                        frame "3" {
                        }
                        frame "4" {
                        }
                        frame "5" {
                        }
                        frame "6" {
                        }
                        frame "7" {
                        }
                        frame "8" {
                        }
                        frame "9" {
                        }
                        frame "10" {
                        }
                        frame "11" {
                        }
                        frame "12" {
                        }
                        frame "13" {
                        }
                        frame "14" {
                        }
                        frame "15" {
                        }
                        frame "16" {
                        }
                        frame "17" {
                        }
                        frame "18" {
                        }
                        frame "19" {
                        }
                        frame "20" {
                        }
                      }
                      n496 = case shown="True" w744 {
                        tunnel: w745 -> [_ w751]
                        tunnel: w742 -> [w746 w747]
                        tunnel: [w746 w747] -> w741
                        frame False {
                        }
                        frame True {
                          # "Loads an open sequence file in the sequence array"
                          n497 = call-poly <vilib>:"Read From Spreadsheet File.vi"("file path (dialog if empty)"=w751) -> ("all rows"=w749:string[][])  [unwired: 6 in, 4 out]
                          n498 = local read "sequence"() -> (w748:string[][])
                          n499 = Build Array (concatenate)(w748, w749) -> (w750:string[][])
                          n500 = local write "sequence"(w750) -> ()
                        }
                      }
                      n501 = local write "path Selection"(w741) -> ()
                    }
                  }
                  frame #2 {
                    w821 = "0" ("Element")
                    n502 = local read "sequence"() -> (w823:string[][])
                    n503 = Build Array("set speed", "20") -> (w815:string[])
                    n504 = Build Array("go straight to coordinates", w821, "0" ("Element"), w821) -> (w818:string[])
                    n505 = Build Array (concatenate)(w823, w815, w818) -> (w822:string[][])
                    n506 = local write "sequence"(w822) -> ()
                  }
                }
              }
              frame "read" {
                n507 = local read "Port ED32i"() -> (w839:refnum<visa-resource-name>)
                n508 = for {
                  N: 3 -> [_]
                  tunnel: [w843] -> w841 mode=indexing
                  i -> [w845]
                  n509 = local read "current coordinates"() -> (w846:T7)
                  n510 = Cluster To Array(cluster=w846) -> (array=w844:dbl[])
                  n511 = Index Array(array=w844, index=w845) -> (element=w843:dbl)
                }
                n512 = call "Serielle Schnittstelle sensor.vi"("Verzögerung vor dem Lesen (ms)"=30, "Write"="xs", "Baudrate"=115200, "VISA-Ressourcenname"=w839) -> ("Read"=w831:string)  [unwired: 7 in]
                n513 = local write "KMT Output"(w831) -> ()
                n514 = Spreadsheet String To Array(delimiter (Tab)=" ", format string="%s", spreadsheet string=w831, array type (2D Dbl)=dbl[] []) -> (array=w830:dbl[])
                n515 = Number To Fractional String(number=w841) -> (F-format string=w834:string[])  [unwired: 3 in]
                n516 = Number To Fractional String(number=w830) -> (F-format string=w833:string[])  [unwired: 3 in]
                n517 = local read "sensor log"() -> (w836:string[][])
                n518 = Build Array (concatenate)(w834, w833) -> (w837:string[])
                n519 = Build Array (concatenate)(w836, w837) -> (w835:string[][])
                n520 = local write "sensor log"(w835) -> ()
              }
              frame "sensor run constant read" {
                # "out an automated reading\nmade in the ongoing data from the sensor\nwas added and the table\nBe \"sensor log\" saved. about\nthe comparison of two timer is the\nelapsed time of the sensor output\nassigned."
                n521 = Tick Count (ms)() -> (millisecond timer value=w849:u32)
                n522 = while {
                  tunnel: w849 -> [w860]
                  stop <- w854 continue-if-true
                  n523 = local read "Port ED33"() -> (w870:refnum<visa-resource-name>)
                  n524 = call "Serielle Schnittstelle sensor.vi"("Verzögerung vor dem Lesen (ms)"=30, "Write"="os", "Baudrate"=115200, "VISA-Ressourcenname"=w870) -> ("Read"=w865:string)  [unwired: 7 in]
                  n525 = Tick Count (ms)() -> (millisecond timer value=w861:u32)
                  n526 = Spreadsheet String To Array(delimiter (Tab)=" ", format string="%s", spreadsheet string=w865, array type (2D Dbl)=dbl[] []) -> (array=w868:dbl[])
                  n527 = Subtract(x=w861, y=w860) -> (x-y=w859:u32)
                  n528 = Number To Fractional String(number=w859, precision (6)=i16 0 ("Genauigkeit (6)")) -> (F-format string=w858:string)  [unwired: 2 in]
                  n529 = Number To Fractional String(number=w868, precision (6)=i16 0 ("Genauigkeit (6)")) -> (F-format string=w862:string[])  [unwired: 2 in]
                  n530 = Build Array (concatenate)(w858, w862) -> (w855:string[])
                  "Array" <- w855
                  n531 = local read "sensor log"() -> (w864:string[][])
                  n532 = Build Array (concatenate)(w864, w855) -> (w863:string[][])
                  n533 = local write "sensor log"(w863) -> ()
                  n534 = local read "ED33reading"() -> (w854:bool)
                }
                n535 = flat-sequence {
                  tunnel: w853 -> [w877]
                  tunnel: w852 -> [w881]
                  tunnel: [w876] -> w851
                  tunnel: [w874] -> w847
                  tunnel: [w887] -> w850
                  tunnel: w851 -> [w887]
                  frame #0 {
                    w880 = cluster{dbl, dbl, dbl, dbl, dbl, dbl, dbl} {0.0, 0.0, 0.0, 0.0, 0.0, 0.0, 0.0}  # zero coordinates
                    n536 = local write "ED33reading"(TRUE) -> ()
                    n537 = local read "Movement"() -> (w879:dbl[])
                    n538 = Bundle(1, 1, 0) -> (w878:cluster{i32, i32, i32})  [unwired: 1 in]
                    n539 = call <userlib>:"SubVI_Multi_linear_interpolation_IF5_IF6.vi"("new position"=w879, "error in"=w877, "coordinates in IF6"=w880, "speed"=w878, "VISA resource name in"=w881) -> ("error out"=w876:errorcluster, "coordinates out IF6"=w875:T16, "VISA resource name in 2"=w874:refnum<visa-resource-name>)  [unwired: 1 in]
                    n540 = local write "current coordinates"(w875) -> ()
                  }
                  frame #1 {
                    n541 = local write "ED33reading"(FALSE) -> ()
                  }
                }
              }
              frame "ED33" {
                # "Approximately equivalent of the \"sensor-run constant read\", only with the untershied that the\ndetection of the elapsed time and the position during reading, the signal of a\nEd33 is evaluated"
                n542 = flat-sequence {
                  tunnel: w894 -> [w911]
                  tunnel: [w911] -> w891
                  tunnel: [w936] -> w892
                  tunnel: w891 -> [w936]
                  tunnel: w890 -> [w943]
                  tunnel: w896 -> [w942]
                  tunnel: [w941] -> w893
                  tunnel: w892 -> [w940]
                  tunnel: [w938] -> w888
                  tunnel: [w1053] -> w895
                  tunnel: w893 -> [w1053]
                  frame #0 {
                    n543 = local read "Mess Zähler"() -> (w898:dbl)
                    n544 = local write "Messsensor"("ED32i" ("Messsensor")) -> ()
                    n545 = Increment(x=w898) -> (x+1=→"Mess Zähler":dbl)
                    n546 = local read "sequence active?"() -> (w910:bool)
                    n547 = case shown="True" w910 {
                      tunnel: [w913 w926] -> w901
                      frame False {
                        n548 = local read "Movement"() -> (w924:dbl[])
                        n549 = local read "Distances"() -> (w922:T5)
                        n550 = Array To Cluster(array=w924) -> (cluster=w923:T22)
                        n551 = Unbundle(w923) -> ("Movement[0]"=w921:dbl, "Movement[1]"=w920:dbl, "Movement[2]"=w919:dbl, "Movement[6]"=w914:dbl, "Movement[7]"=w915:dbl, "Movement[8]"=w912:dbl)  [unwired: 3 out]
                        n552 = Unbundle(w922) -> ("X-Abstand (0)"=w918:sgl, "Y-Abstand (0)"=w917:sgl, "Z-Abstand (0)"=w916:sgl)
                        n553 = Bundle("Movement[0]"=w921, "Movement[1]"=w920, "Movement[2]"=w919, "X-Abstand (0)"=w918, "Y-Abstand (0)"=w917, "Z-Abstand (0)"=w916, "Movement[6]"=w914, "Movement[7]"=w915, "Movement[8]"=w912) -> (w913:T23)  [unwired: 1 in]
                      }
                      frame True {
                        n554 = for {
                          N: 7 -> [_]
                          tunnel: [w928] -> w925 mode=indexing
                          i -> [w930]
                          n555 = local read "current sequence"() -> (w933:string[])
                          n556 = Add(x=1.0, y=w930) -> (x+y=w932:dbl)
                          n557 = Index Array(array=w933, index=w932) -> (element=w929:string)
                          n558 = Fract/Exp String To Number(string=w929) -> (number=w928:dbl)  [unwired: 3 in, 1 out]
                        }
                        n559 = Array To Cluster(array=w925) -> (cluster=w926:T21)
                      }
                    }
                    n560 = Unbundle(w901) -> ("[0]"=w897:dbl, "[1]"=w909:dbl, "[2]"=w908:dbl, "[3]"=w905:dbl, "[4]"=w904:dbl, "[5]"=w903:dbl)  [unwired: 3 out]
                    n561 = Bundle("[0]"=w897, "[1]"=w909, "[2]"=w908) -> (w907:cluster{"[0]":dbl, "[1]":dbl, "[2]":dbl})  [unwired: 1 in]
                    n562 = Bundle("[3]"=w905, "[4]"=w904, "[5]"=w903) -> (w902:cluster{"[3]":dbl, "[4]":dbl, "[5]":dbl})  [unwired: 1 in]
                    n563 = local write "Distances"(w902) -> ()
                    n564 = Cluster To Array(cluster=w907) -> (array=w906:dbl[])
                    n565 = local write "Movement"(w906) -> ()
                  }
                  frame #1 {
                    n566 = local write "ED33reading"(TRUE ("reading")) -> ()
                    n567 = local read "current coordinates"() -> (→"Measurement start value":T7)
                  }
                  frame #2 {
                    w951 = u32 10000  # timeout (10sec)
                    n568 = local read "Port ED32i"() -> (w944:refnum<visa-resource-name>)
                    n569 = call-poly "VISA Configure Serial Port"("VISA resource name"=w944, "timeout (10sec)"=w951, "baud rate (9600)"="baud rate (9600)", "data bits (8)"="data bits", "parity (0:none)"="parity", "stop bits (10: 1 bit)"="stop bits") -> ("VISA resource name out"=w947:refnum<visa-resource-name>, "error out"=w949:errorcluster)  [unwired: 3 in, 5 out]
                    n570 = call-poly "VISA Configure Serial Port"("VISA resource name"=w943, "timeout (10sec)"=w951, "baud rate (9600)"="baud rate", "data bits (8)"="data bits", "parity (0:none)"="parity", "error in (no error)"=w949, "stop bits (10: 1 bit)"="stop bits", "flow control (0:none)"="flow control") -> ("VISA resource name out"=w957:refnum<visa-resource-name>, "error out"=w958:errorcluster)  [unwired: 1 in, 5 out]
                    n571 = while {
                      tunnel: w958 -> [w971]
                      tunnel: w957 -> [w970]
                      tunnel: [w969] -> w956
                      tunnel: [w968] -> w955
                      tunnel: w947 -> [w967]
                      tunnel: [w966] -> w939
                      tunnel: [w965] -> w945
                      tunnel: w942 -> [w960]
                      tunnel: [w963] -> w941
                      tunnel: w940 -> [w962]
                      tunnel: [w961] -> w938
                      stop <- w964 continue-if-true
                      n572 = stacked-sequence {
                        tunnel: w971 -> [w1012 _ _]
                        tunnel: w970 -> [w1011 _ _]
                        tunnel: [w973 _ _] -> w969
                        tunnel: [w1010 _ _] -> w968
                        tunnel: w967 -> [w1004 _ _]
                        tunnel: [w999 _ _] -> w966
                        tunnel: [w998 _ _] -> w965
                        tunnel: [_ w1034 _] -> w963
                        tunnel: w962 -> [_ w1033 _]
                        tunnel: [_ w1032 _] -> w961
                        tunnel: w960 -> [_ w1031 _]
                        frame #0 {
                          # "Specified number of bytes is read."
                          n573 = case shown="True" TRUE {
                            tunnel: [w1018 w1029] -> w1009
                            tunnel: w1011 -> [w1020 w1028]
                            tunnel: w1012 -> [w1018 w1024]
                            tunnel: [w1020 w1027] -> w1008
                            tunnel: "write 3" -> [_ w1026]
                            tunnel: w1004 -> [w1019 w1025]
                            tunnel: [w1019 w1023] -> w1003
                            tunnel: [w1018 w1022] -> w1002
                            tunnel: "write 2" -> [_ w1021]
                            frame False {
                            }
                            frame True {
                              # "Send bytes to port."
                              n574 = VISA Write(VISA resource name=w1028, write buffer=w1026, error in (no error)=w1024) -> (VISA resource name out=w1027:refnum<visa-resource-name>, error out=w1029:errorcluster)  [unwired: 1 out]
                              n575 = VISA Write(VISA resource name=w1025, write buffer=w1021, error in (no error)=w1024) -> (VISA resource name out=w1023:refnum<visa-resource-name>, error out=w1022:errorcluster)  [unwired: 1 out]
                            }
                          }
                          n576 = stacked-sequence {
                            tunnel: w1009 -> [w1017]
                            tunnel: [w1017] -> w1005
                            tunnel: w1008 -> [w1016]
                            tunnel: [w1016] -> w1006
                            tunnel: w1003 -> [w1014]
                            tunnel: w1002 -> [w1013]
                            tunnel: [w1014] -> w1001
                            tunnel: [w1013] -> w1000
                            frame #0 {
                              n577 = Wait (ms)(milliseconds to wait="delay before read (ms)") -> ()  [unwired: 1 out]
                            }
                          }
                          n578 = property class="Instr"(reference=w1006, error in=w1005) -> (reference out=w997:refnum<visa-resource-name>, error out=w996:errorcluster, "Serial Settings:Number of Bytes at Serial Port"=w972:u32)
                          "bytes read" <- w972
                          n579 = property class="Instr"(reference=w1001, error in=w1000) -> (reference out=w995:refnum<visa-resource-name>, error out=w994:errorcluster, "Serial Settings:Number of Bytes at Serial Port"=w993:u32)
                          "Serial Settings:Number of Bytes at Serial Port" <- w993
                          n580 = VISA Read(VISA resource name=w995, byte count=w993, error in (no error)=w994) -> (VISA resource name out=w998:refnum<visa-resource-name>, read buffer=w985:string, error out=w999:errorcluster)  [unwired: 1 out]
                          n581 = VISA Read(VISA resource name=w997, byte count=w972, error in (no error)=w996) -> (VISA resource name out=w1010:refnum<visa-resource-name>, read buffer=w986:string, error out=w973:errorcluster)  [unwired: 1 out]
                          n582 = call "ED33-32i-1.3(SubVI).vi"("read buffer"=w986, "read buffer 2"=w985) -> ("Teil-String"=w983:string, "Teil-String 2"=w982:string, "Teil-String 3"=w981:string, "Teil-String 4"=w980:string, "Teil-String 5"=w979:string, "read string"=→"read string 2":string, "Teil-String 6"=w978:string, "Teil-String 7"=w977:string, "read string 2"=→"read string":string, "Teil-String 8"=w976:string, "Zeit"=w984:string, "Länge 1"=w974:string)  [unwired: 4 in, 2 out]
                          n583 = Build Array(w974, w984, w983, w982, w981, w980, w979, w978, w977, w976) -> (w990:string[])
                          n584 = local read "Attached Array"() -> (w987:string[][])
                          n585 = Build Array (concatenate)(w990, w987) -> (→"Attached Array":string[][])
                        }
                        frame #1 {
                          n586 = Bundle(1, 1, 1) -> (w1038:cluster{i32, i32, i32})  [unwired: 1 in]
                          n587 = call <userlib>:"SubVI_Geradeninterpolation_3_Achs_IF5_IF6.vi"("VISA resource name in"=w1031, "Geschwindigkeiten"=w1038, "IF5=F/IF6=T\n(IF6=T) in"=TRUE ("IF5=F/IF6=T\n(IF6=T) in"), "Abstände"="Distances", "error in"=w1033, "Richtungen"="Direction 2") -> ("VISA resource name out"=w1034:refnum<visa-resource-name>, "Koordinaten IF6"=w1043:T16, "error out"=w1032:errorcluster)  [unwired: 4 in, 3 out]
                          n588 = local write "current coordinates"(w1043) -> ()
                          n589 = local read "Measurement start value"() -> (w1045:T7)
                          n590 = Unbundle(w1043) -> ("Schritte Y"=w1044:sgl)  [unwired: 6 out]
                          n591 = local read "Movement"() -> (w1030:dbl[])
                          n592 = Unbundle(w1045) -> ("steps y"=w1046:dbl)  [unwired: 6 out]
                          n593 = Array To Cluster(array=w1030) -> (cluster=w1042:T22)
                          n594 = Subtract(x=w1044, y=w1046) -> (x-y=w1048:dbl)
                          n595 = Unbundle(w1042) -> ("Movement[1]"=w1047:dbl)  [unwired: 8 out]
                          n596 = Greater Or Equal?(x=w1048, y=w1047) -> (x >= y?=w1049:bool)
                          n597 = case shown="True" w1049 {
                            frame False {
                            }
                            frame True {
                              n598 = local write "ED33reading"(FALSE) -> ()
                            }
                          }
                        }
                        frame #2 {
                          n599 = Wait (ms)(milliseconds to wait=u32 100 ("Zu wartende ms")) -> ()  [unwired: 1 out]
                        }
                      }
                      n600 = local read "ED33reading"() -> (w964:bool)
                    }
                    n601 = VISA Close(VISA resource name=w955, error in (no error)=w956) -> (error out=w954:errorcluster)
                    n602 = VISA Close(VISA resource name=w945, error in (no error)=w939) -> (error out=w946:errorcluster)
                    n603 = call <vilib>:"Simple Error Handler.vi"("error in (no error)"=w954) -> ()  [unwired: 1 in, 8 out]
                    n604 = call <vilib>:"Simple Error Handler.vi"("error in (no error)"=w946) -> ()  [unwired: 1 in, 8 out]
                  }
                  frame #3 {
                    n605 = local write "key stm"("auto" ("key stm")) -> ()
                  }
                }
                n606 = local read "Port ED33"() -> (w890:refnum<visa-resource-name>)
              }
              frame "KMT" {
                # "Approximately equivalent of the \"sensor-run constant read\", only with the untershied that the\ndetection of the elapsed time and the position during reading, the signal of a\nEd33 is evaluated"
                n607 = flat-sequence {
                  tunnel: w1059 -> [w1077]
                  tunnel: [w1077] -> w1056
                  tunnel: [w1103] -> w1062
                  tunnel: w1056 -> [w1103]
                  tunnel: w1060 -> [w1111]
                  tunnel: w1058 -> [w1110]
                  tunnel: [w1109] -> w1061
                  tunnel: w1062 -> [w1108]
                  tunnel: [w1104] -> w1054
                  tunnel: [w1221] -> w1057
                  tunnel: w1061 -> [w1221]
                  frame #0 {
                    n608 = local read "Mess Zähler"() -> (w1063:dbl)
                    n609 = local read "sequence active?"() -> (w1076:bool)
                    n610 = case shown="True" w1076 {
                      tunnel: [w1079 w1092] -> w1066
                      frame False {
                        n611 = local read "Movement"() -> (w1090:dbl[])
                        n612 = local read "Distances"() -> (w1088:T5)
                        n613 = Array To Cluster(array=w1090) -> (cluster=w1089:T22)
                        n614 = Unbundle(w1088) -> ("X-Abstand (0)"=w1084:sgl, "Y-Abstand (0)"=w1083:sgl, "Z-Abstand (0)"=w1082:sgl)
                        n615 = Unbundle(w1089) -> ("Movement[0]"=w1087:dbl, "Movement[1]"=w1086:dbl, "Movement[2]"=w1085:dbl, "Movement[6]"=w1080:dbl, "Movement[7]"=w1081:dbl, "Movement[8]"=w1078:dbl)  [unwired: 3 out]
                        n616 = Bundle("Movement[0]"=w1087, "Movement[1]"=w1086, "Movement[2]"=w1085, "X-Abstand (0)"=w1084, "Y-Abstand (0)"=w1083, "Z-Abstand (0)"=w1082, "Movement[6]"=w1080, "Movement[7]"=w1081, "Movement[8]"=w1078) -> (w1079:T23)  [unwired: 1 in]
                      }
                      frame True {
                        n617 = for {
                          N: 7 -> [_]
                          tunnel: [w1094] -> w1091 mode=indexing
                          i -> [w1096]
                          n618 = local read "current sequence"() -> (w1099:string[])
                          n619 = Add(x=1.0, y=w1096) -> (x+y=w1098:dbl)
                          n620 = Index Array(array=w1099, index=w1098) -> (element=w1095:string)
                          n621 = Fract/Exp String To Number(string=w1095) -> (number=w1094:dbl)  [unwired: 3 in, 1 out]
                        }
                        n622 = Array To Cluster(array=w1091) -> (cluster=w1092:T21)
                      }
                    }
                    n623 = Increment(x=w1063) -> (x+1=w1064:dbl)
                    n624 = local write "Mess Zähler"(w1064) -> ()
                    n625 = Unbundle(w1066) -> ("[0]"=w1075:dbl, "[1]"=w1074:dbl, "[2]"=w1073:dbl, "[3]"=w1070:dbl, "[4]"=w1069:dbl, "[5]"=w1068:dbl)  [unwired: 3 out]
                    n626 = Bundle("[0]"=w1075, "[1]"=w1074, "[2]"=w1073) -> (w1072:cluster{"[0]":dbl, "[1]":dbl, "[2]":dbl})  [unwired: 1 in]
                    n627 = Bundle("[3]"=w1070, "[4]"=w1069, "[5]"=w1068) -> (w1067:cluster{"[3]":dbl, "[4]":dbl, "[5]":dbl})  [unwired: 1 in]
                    n628 = local write "Distances"(w1067) -> ()
                    n629 = Cluster To Array(cluster=w1072) -> (array=w1071:dbl[])
                    n630 = local write "Movement"(w1071) -> ()
                    "Messsensor" <- "KMT"
                  }
                  frame #1 {
                    n631 = local write "KMT read"(TRUE ("reading")) -> ()
                    n632 = local write "KMT read start"(FALSE ("KMT read start")) -> ()
                    n633 = local read "current coordinates"() -> (w1101:T7)
                    n634 = local write "Measurement start value"(w1101) -> ()
                  }
                  frame #2 {
                    w1119 = u32 10000  # timeout (10sec)
                    n635 = call-poly "VISA Configure Serial Port"("VISA resource name"="KMT Port", "timeout (10sec)"=w1119, "baud rate (9600)"="baud rate (9600) 2", "data bits (8)"="data bits 6", "parity (0:none)"="parity 6", "stop bits (10: 1 bit)"="stop bits 6") -> ("VISA resource name out"=w1114:refnum<visa-resource-name>, "error out"=w1116:errorcluster)  [unwired: 3 in, 5 out]
                    n636 = call-poly "VISA Configure Serial Port"("VISA resource name"=w1111, "timeout (10sec)"=w1119, "baud rate (9600)"="baud rate 6", "data bits (8)"="data bits 6", "parity (0:none)"="parity 6", "error in (no error)"=w1116, "stop bits (10: 1 bit)"="stop bits 6", "flow control (0:none)"="flow control 6") -> ("VISA resource name out"=w1124:refnum<visa-resource-name>, "error out"=w1125:errorcluster)  [unwired: 1 in, 5 out]
                    n637 = while {
                      tunnel: w1125 -> [w1138]
                      tunnel: w1124 -> [w1137]
                      tunnel: [w1136] -> w1123
                      tunnel: [w1135] -> w1122
                      tunnel: w1114 -> [w1134]
                      tunnel: [w1133] -> w1107
                      tunnel: [w1132] -> w1112
                      tunnel: w1110 -> [w1127]
                      tunnel: [w1130] -> w1109
                      tunnel: w1108 -> [w1129]
                      tunnel: [w1128] -> w1104
                      stop <- w1131 continue-if-true
                      n638 = stacked-sequence {
                        tunnel: w1138 -> [w1179 _ _]
                        tunnel: w1137 -> [w1178 _ _]
                        tunnel: [w1177 _ _] -> w1136
                        tunnel: [w1176 _ _] -> w1135
                        tunnel: w1134 -> [w1171 _ _]
                        tunnel: [w1166 _ _] -> w1133
                        tunnel: [w1165 _ _] -> w1132
                        tunnel: [_ w1202 _] -> w1130
                        tunnel: w1129 -> [_ w1201 _]
                        tunnel: [_ w1200 _] -> w1128
                        tunnel: w1127 -> [_ w1199 _]
                        frame #0 {
                          # "Length 2 is on: The means Renishaw measurement values are Captures !!!!!!!!!"
                          # "Angegebene Anzahl an Bytes wird gelesen."
                          n639 = case shown="True" TRUE {
                            tunnel: [w1185 w1196] -> w1175
                            tunnel: w1178 -> [w1187 w1195]
                            tunnel: w1179 -> [w1185 w1191]
                            tunnel: [w1187 w1194] -> w1139
                            tunnel: "write ED33" -> [_ w1193]
                            tunnel: w1171 -> [w1186 w1192]
                            tunnel: [w1186 w1190] -> w1170
                            tunnel: [w1185 w1189] -> w1169
                            tunnel: "write KMT" -> [_ w1188]
                            frame False {
                            }
                            frame True {
                              # "Bytes an Port senden."
                              n640 = VISA Write(VISA resource name=w1192, write buffer=w1188, error in (no error)=w1191) -> (VISA resource name out=w1190:refnum<visa-resource-name>, error out=w1189:errorcluster)  [unwired: 1 out]
                              n641 = VISA Write(VISA resource name=w1195, write buffer=w1193, error in (no error)=w1191) -> (VISA resource name out=w1194:refnum<visa-resource-name>, error out=w1196:errorcluster)  [unwired: 1 out]
                            }
                          }
                          n642 = stacked-sequence {
                            tunnel: w1175 -> [w1184]
                            tunnel: [w1184] -> w1172
                            tunnel: w1139 -> [w1183]
                            tunnel: [w1183] -> w1173
                            tunnel: w1170 -> [w1180]
                            tunnel: w1169 -> [w1181]
                            tunnel: [w1180] -> w1168
                            tunnel: [w1181] -> w1167
                            frame #0 {
                              n643 = Wait (ms)(milliseconds to wait="delay before read (ms) 6") -> ()  [unwired: 1 out]
                            }
                          }
                          n644 = property class="Instr"(reference=w1168, error in=w1167) -> (reference out=w1162:refnum<visa-resource-name>, error out=w1161:errorcluster, "Serial Settings:Number of Bytes at Serial Port"=w1160:u32)
                          n645 = property class="Instr"(reference=w1173, error in=w1172) -> (reference out=w1164:refnum<visa-resource-name>, error out=w1163:errorcluster, "Serial Settings:Number of Bytes at Serial Port"=w1157:u32)
                          "bytes read 6" <- w1157
                          n646 = VISA Read(VISA resource name=w1162, byte count=w1160, error in (no error)=w1161) -> (VISA resource name out=w1165:refnum<visa-resource-name>, read buffer=w1141:string, error out=w1166:errorcluster)  [unwired: 1 out]
                          n647 = VISA Read(VISA resource name=w1164, byte count=w1157, error in (no error)=w1163) -> (VISA resource name out=w1176:refnum<visa-resource-name>, read buffer=w1142:string, error out=w1177:errorcluster)  [unwired: 1 out]
                          n648 = call "KMT_decoder1.0.vi"("read buffer"=w1142, "read buffer 2"=w1141) -> ("Teil-String"=w1151:string, "Teil-String 2"=w1150:string, "Teil-String 3"=w1149:string, "Teil-String 4"=w1148:string, "Teil-String 5"=w1147:string, "read string"=→"read string 5":string, "Teil-String 6"=w1146:string, "Teil-String 7"=w1145:string, "read string 2"=→"read string 6":string, "Teil-String 8"=w1144:string, "Zeit"=w1152:string, "Länge 2"=w1140:string)  [unwired: 4 in, 2 out]
                          n649 = local read "Attached Array"() -> (w1156:string[][])
                          n650 = Build Array(w1140, w1152, w1151, w1150, w1149, w1148, w1147, w1146, w1145, w1144) -> (w1143:string[])
                          n651 = Build Array (concatenate)(w1156, w1143) -> (w1155:string[][])
                          n652 = local write "Attached Array"(w1155) -> ()
                        }
                        frame #1 {
                          n653 = local read "Direction 2"() -> (w1198:T6)
                          n654 = local read "Distances"() -> (w1197:T5)
                          n655 = local read "Measurement start value"() -> (w1212:T7)
                          n656 = Bundle(1, 1, 1) -> (w1206:cluster{i32, i32, i32})  [unwired: 1 in]
                          n657 = local read "Movement"() -> (w1208:dbl[])
                          n658 = call "SubVI_Geradeninterpolation_3_Achs_IF5_IF6 - Kopie.vi"("VISA resource name in"=w1199, "Geschwindigkeiten"=w1206, "IF5=F/IF6=T\n(IF6=T) in"=TRUE ("IF5=F/IF6=T\n(IF6=T) in"), "Abstände"=w1197, "error in"=w1201, "Richtungen"=w1198) -> ("VISA resource name out"=w1202:refnum<visa-resource-name>, "Koordinaten IF6"=w1210:T16, "error out"=w1200:errorcluster)  [unwired: 4 in, 3 out]
                          n659 = Array To Cluster(array=w1208) -> (cluster=w1209:T22)
                          n660 = Unbundle(w1212) -> ("steps y"=w1213:dbl)  [unwired: 6 out]
                          n661 = Unbundle(w1210) -> ("Schritte Y"=w1211:sgl)  [unwired: 6 out]
                          n662 = local write "current coordinates"(w1210) -> ()
                          n663 = Subtract(x=w1211, y=w1213) -> (x-y=w1215:dbl)
                          n664 = Unbundle(w1209) -> ("Movement[1]"=w1214:dbl)  [unwired: 8 out]
                          n665 = Greater Or Equal?(x=w1215, y=w1214) -> (x >= y?=w1216:bool)
                          n666 = case shown="True" w1216 {
                            frame False {
                            }
                            frame True {
                              n667 = local write "KMT read"(FALSE) -> ()
                            }
                          }
                        }
                        frame #2 {
                          n668 = Wait (ms)(milliseconds to wait=u32 100 ("Zu wartende ms")) -> ()  [unwired: 1 out]
                        }
                      }
                      n669 = local read "KMT read"() -> (w1131:bool)
                    }
                    n670 = VISA Close(VISA resource name=w1112, error in (no error)=w1107) -> (error out=w1113:errorcluster)
                    n671 = VISA Close(VISA resource name=w1122, error in (no error)=w1123) -> (error out=w1121:errorcluster)
                    n672 = call <vilib>:"Simple Error Handler.vi"("error in (no error)"=w1113) -> ()  [unwired: 1 in, 8 out]
                    n673 = call <vilib>:"Simple Error Handler.vi"("error in (no error)"=w1121) -> ()  [unwired: 1 in, 8 out]
                  }
                  frame #3 {
                    n674 = local write "KMT read start"(FALSE ("KMT read start")) -> ()
                    n675 = local write "key stm"("auto" ("key stm")) -> ()
                  }
                }
                n676 = local read "Port ED33"() -> (w1060:refnum<visa-resource-name>)
              }
              frame "GAUS" {
                n677 = flat-sequence {
                  tunnel: w1226 -> [w1231]
                  tunnel: [w1231] -> w1227
                  tunnel: w1223 -> [_]
                  tunnel: [w1268] -> w1228
                  tunnel: w1227 -> [w1268]
                  tunnel: [w1287] -> w1229
                  tunnel: w1228 -> [w1282]
                  tunnel: w1223 -> [w1285]
                  tunnel: [w1284] -> w1225
                  tunnel: [w1375] -> w1230
                  tunnel: w1229 -> [w1375]
                  tunnel: [w1374] -> w1222
                  tunnel: w1225 -> [w1374]
                  frame #0 {
                    n678 = local read "Mess Zähler"() -> (w1244:dbl)
                    n679 = local write "Messsensor"("GAUS" ("Messsensor")) -> ()
                    n680 = local read "sequence active?"() -> (w1242:bool)
                    n681 = Increment(x=w1244) -> (x+1=w1243:dbl)
                    n682 = local write "Mess Zähler"(w1243) -> ()
                    n683 = case shown="True" w1242 {
                      tunnel: [w1246 w1259] -> w1236
                      frame False {
                        n684 = local read "Movement"() -> (w1248:dbl[])
                        n685 = local read "Distances"() -> (w1249:T5)
                        n686 = Array To Cluster(array=w1248) -> (cluster=w1247:T22)
                        n687 = Unbundle(w1247) -> ("Movement[0]"=w1258:dbl, "Movement[1]"=w1257:dbl, "Movement[2]"=w1256:dbl, "Movement[6]"=w1251:dbl, "Movement[7]"=w1252:dbl, "Movement[8]"=w1250:dbl)  [unwired: 3 out]
                        n688 = Unbundle(w1249) -> ("X-Abstand (0)"=w1255:sgl, "Y-Abstand (0)"=w1254:sgl, "Z-Abstand (0)"=w1253:sgl)
                        n689 = Bundle("Movement[0]"=w1258, "Movement[1]"=w1257, "Movement[2]"=w1256, "X-Abstand (0)"=w1255, "Y-Abstand (0)"=w1254, "Z-Abstand (0)"=w1253, "Movement[6]"=w1251, "Movement[7]"=w1252, "Movement[8]"=w1250) -> (w1246:T23)  [unwired: 1 in]
                      }
                      frame True {
                        n690 = for {
                          N: 7 -> [_]
                          tunnel: [w1263] -> w1260 mode=indexing
                          i -> [w1262]
                          n691 = local read "current sequence"() -> (w1264:string[])
                          n692 = Add(x=1.0, y=w1262) -> (x+y=w1267:dbl)
                          n693 = Index Array(array=w1264, index=w1267) -> (element=w1265:string)
                          n694 = Fract/Exp String To Number(string=w1265) -> (number=w1263:dbl)  [unwired: 3 in, 1 out]
                        }
                        n695 = Array To Cluster(array=w1260) -> (cluster=w1259:T21)
                      }
                    }
                    n696 = Unbundle(w1236) -> ("[0]"=w1235:dbl, "[1]"=w1241:dbl, "[2]"=w1240:dbl, "[3]"=w1239:dbl, "[4]"=w1238:dbl, "[5]"=w1237:dbl)  [unwired: 3 out]
                    n697 = Bundle("[0]"=w1235, "[1]"=w1241, "[2]"=w1240) -> (w1234:cluster{"[0]":dbl, "[1]":dbl, "[2]":dbl})  [unwired: 1 in]
                    n698 = Bundle("[3]"=w1239, "[4]"=w1238, "[5]"=w1237) -> (w1232:cluster{"[3]":dbl, "[4]":dbl, "[5]":dbl})  [unwired: 1 in]
                    n699 = local write "Distances"(w1232) -> ()
                    n700 = Cluster To Array(cluster=w1234) -> (array=w1233:dbl[])
                    n701 = local write "Movement"(w1233) -> ()
                  }
                  frame #1 {
                    n702 = local write "GAUS read strart 2"(FALSE ("GAUS read start")) -> ()
                    n703 = local read "current coordinates"() -> (w1270:T7)
                    n704 = local write "Measurement start value"(w1270) -> ()
                    "GAUS read" <- TRUE ("GAUS read")
                  }
                  frame #2 {
                    n705 = call-poly "VISA Configure Serial Port"("VISA resource name"="GAUS Port", "baud rate (9600)"="baud rate (9600) 3", "error in (no error)"=w1282) -> ("VISA resource name out"=w1281:refnum<visa-resource-name>, "error out"=w1272:errorcluster)  [unwired: 11 in]
                    n706 = local read "Port ED33"() -> (w1280:refnum<visa-resource-name>)
                    n707 = call-poly "VISA Configure Serial Port"("VISA resource name"=w1280, "baud rate (9600)"="baud rate (9600) 4", "error in (no error)"=w1272) -> ("VISA resource name out"=w1278:refnum<visa-resource-name>, "error out"=w1277:errorcluster)  [unwired: 11 in]
                    n708 = while {
                      tunnel: w1281 -> [w1299]
                      tunnel: [w1298] -> w1288
                      tunnel: w1277 -> [w1297]
                      tunnel: [w1293] -> w1287
                      tunnel: [w1296] -> w1286
                      tunnel: w1285 -> [w1295]
                      tunnel: [w1294] -> w1284
                      tunnel: w1278 -> [w1292]
                      tunnel: [w1291] -> w1275
                      tunnel: [w1290] -> w1274
                      stop <- w1300 continue-if-true
                      n709 = stacked-sequence {
                        tunnel: w1299 -> [w1317 _]
                        tunnel: [w1321 _] -> w1298
                        tunnel: w1297 -> [w1315 w1355]
                        tunnel: [w1320 _] -> w1296
                        tunnel: w1295 -> [_ w1356]
                        tunnel: [_ w1354] -> w1294
                        tunnel: [_ w1353] -> w1293
                        tunnel: w1292 -> [w1314 _]
                        tunnel: [w1306 _] -> w1291
                        tunnel: [w1305 _] -> w1290
                        frame #0 {
                          n710 = local read "write ED33"() -> (w1313:string)
                          n711 = case shown="True" TRUE {
                            tunnel: [w1340 w1351] -> w1334
                            tunnel: w1317 -> [w1342 w1350]
                            tunnel: w1315 -> [w1340 w1346]
                            tunnel: [w1342 w1349] -> w1333
                            tunnel: "string to write 2" -> [_ w1348]
                            tunnel: w1314 -> [w1341 w1347]
                            tunnel: w1313 -> [_ w1345]
                            tunnel: [w1341 w1344] -> w1312
                            tunnel: [w1340 w1343] -> w1311
                            frame False {
                            }
                            frame True {
                              # "Send bytes to port."
                              n712 = VISA Write(VISA resource name=w1350, write buffer=w1348, error in (no error)=w1346) -> (VISA resource name out=w1349:refnum<visa-resource-name>, error out=w1351:errorcluster)  [unwired: 1 out]
                              n713 = VISA Write(VISA resource name=w1347, write buffer=w1345, error in (no error)=w1346) -> (VISA resource name out=w1344:refnum<visa-resource-name>, error out=w1343:errorcluster)  [unwired: 1 out]
                            }
                          }
                          n714 = stacked-sequence {
                            tunnel: w1334 -> [w1339]
                            tunnel: [w1339] -> w1331
                            tunnel: w1333 -> [w1338]
                            tunnel: [w1338] -> w1332
                            tunnel: [w1336] -> w1310
                            tunnel: w1312 -> [w1336]
                            tunnel: [w1335] -> w1309
                            tunnel: w1311 -> [w1335]
                            frame #0 {
                              n715 = Wait (ms)(milliseconds to wait="delay before read (ms) 7") -> ()  [unwired: 1 out]
                            }
                          }
                          n716 = property class="Instr"(reference=w1332, error in=w1331) -> (reference out=w1330:refnum<visa-resource-name>, error out=w1329:errorcluster, "Serial Settings:Number of Bytes at Serial Port"=w1327:u32)
                          n717 = property class="Instr"(reference=w1310, error in=w1309) -> (reference out=w1308:refnum<visa-resource-name>, error out=w1307:errorcluster, "Serial Settings:Number of Bytes at Serial Port"=w1304:u32)
                          n718 = VISA Read(VISA resource name=w1330, byte count=w1327, error in (no error)=w1329) -> (VISA resource name out=w1321:refnum<visa-resource-name>, read buffer=w1303:string, error out=w1320:errorcluster)  [unwired: 1 out]
                          n719 = VISA Read(VISA resource name=w1308, byte count=w1304, error in (no error)=w1307) -> (VISA resource name out=w1306:refnum<visa-resource-name>, read buffer=w1302:string, error out=w1305:errorcluster)  [unwired: 1 out]
                          n720 = local read "Attached Array"() -> (w1322:string[][])
                          n721 = call "GAUS_decoder1.0.vi"("read buffer"=w1302, "read buffer 2"=w1303) -> ("Ergebnis-String"=w1301:string, "read string"=→"read string 8":string, "read string 2"=→"read string 7":string, "Zeit"=w1325:string, "Länge 1"=w1326:string)  [unwired: 10 in, 3 out]
                          n722 = Build Array(w1326, w1325, w1301) -> (w1324:string[])
                          n723 = Build Array (concatenate)(w1322, w1324) -> (w1323:string[][])
                          n724 = local write "Attached Array"(w1323) -> ()
                        }
                        frame #1 {
                          n725 = local read "Direction 2"() -> (w1358:T6)
                          n726 = local read "Distances"() -> (w1360:T5)
                          n727 = local read "Measurement start value"() -> (w1362:T7)
                          n728 = Bundle(20, 20, 20) -> (w1363:cluster{i32, i32, i32})  [unwired: 1 in]
                          n729 = local read "Movement"() -> (w1361:dbl[])
                          n730 = call "SubVI_Geradeninterpolation_3_Achs_IF5_IF6 - Kopie.vi"("VISA resource name in"=w1356, "Geschwindigkeiten"=w1363, "IF5=F/IF6=T\n(IF6=T) in"=TRUE ("IF5=F/IF6=T\n(IF6=T) in"), "Abstände"=w1360, "error in"=w1355, "Richtungen"=w1358) -> ("VISA resource name out"=w1354:refnum<visa-resource-name>, "Koordinaten IF6"=w1359:T16, "error out"=w1353:errorcluster)  [unwired: 4 in, 3 out]
                          n731 = Array To Cluster(array=w1361) -> (cluster=w1367:T22)
                          n732 = Unbundle(w1362) -> ("steps y"=w1369:dbl)  [unwired: 6 out]
                          n733 = Unbundle(w1359) -> ("Schritte Y"=w1368:sgl)  [unwired: 6 out]
                          n734 = local write "current coordinates"(w1359) -> ()
                          n735 = Subtract(x=w1368, y=w1369) -> (x-y=w1371:dbl)
                          n736 = Unbundle(w1367) -> ("Movement[1]"=w1370:dbl)  [unwired: 8 out]
                          n737 = Greater Or Equal?(x=w1371, y=w1370) -> (x >= y?=w1357:bool)
                          n738 = case shown="True" w1357 {
                            frame False {
                            }
                            frame True {
                              n739 = local write "GAUS read"(FALSE ("GAUS read")) -> ()
                            }
                          }
                        }
                      }
                      n740 = local read "GAUS read"() -> (w1300:bool)
                    }
                    n741 = VISA Close(VISA resource name=w1288, error in (no error)=w1286) -> (error out=w1289:errorcluster)
                    n742 = VISA Close(VISA resource name=w1275, error in (no error)=w1274) -> (error out=w1276:errorcluster)
                    n743 = call <vilib>:"Simple Error Handler.vi"("error in (no error)"=w1289) -> ()  [unwired: 1 in, 8 out]
                    n744 = call <vilib>:"Simple Error Handler.vi"("error in (no error)"=w1276) -> ()  [unwired: 1 in, 8 out]
                  }
                  frame #3 {
                    n745 = local write "GAUS read strart 2"(FALSE ("GAUS read start")) -> ()
                    n746 = local write "key stm"("auto" ("key stm")) -> ()
                  }
                }
              }
              frame "Save as text" {
                w1379 = "" ("String (\"\")")
                w1381 = "_ " ("Name oder relativer Pfad")
                n747 = local read "sequence active?"() -> (w1397:bool)
                n748 = case shown="True" w1397 {
                  tunnel: [string[] [] w1412] -> w1400
                  frame False {
                  }
                  frame True {
                    n749 = for {
                      N: 3 -> [_]
                      tunnel: [w1413] -> w1412 mode=indexing
                      i -> [w1414]
                      n750 = local read "current sequence"() -> (w1417:string[])
                      n751 = Add(x=1.0, y=w1414) -> (x+y=w1416:dbl)
                      n752 = Index Array(array=w1417, index=w1416) -> (element=w1413:string)
                    }
                  }
                }
                n753 = local read "Distances"() -> (w1390:T5)
                n754 = local read "Mess Zähler"() -> (w1380:dbl)
                n755 = local read "Movement"() -> (w1393:dbl[])
                n756 = Unbundle(w1390) -> ("Y-Abstand (0)"=w1391:sgl)  [unwired: 2 out]
                n757 = Array To Cluster(array=w1400) -> (cluster=w1389:T24)
                n758 = Get Date/Time In Seconds() -> (seconds since 1Jan1904=w1385:timestamp)
                n759 = local read "Messsensor"() -> (w1388:string)
                n760 = Array To Cluster(array=w1393) -> (cluster=w1394:T22)
                n761 = Format Value(string ("")=w1379, value (0)=w1380) -> (output string=w1378:string)  [unwired: 1 in]
                n762 = Unbundle(w1389) -> ("[0]"=w1384:string)  [unwired: 8 out]
                n763 = Get Date/Time String(seconds (now)=w1385) -> (date string=w1386:string)  [unwired: 2 in, 1 out]
                n764 = Format Value(string ("")=w1379, value (0)=w1391) -> (output string=w1392:string)  [unwired: 1 in]
                n765 = Unbundle(w1394) -> ("Movement[1]"=w1395:dbl)  [unwired: 8 out]
                n766 = Format Value(string ("")=w1379, value (0)=w1395) -> (output string=w1396:string)  [unwired: 1 in]
                n767 = Concatenate Strings(w1386, w1381, w1388, w1381, w1392, w1381, w1396, w1381, w1384, w1381, w1378, ".txt") -> (w1398:string)
                n768 = Build Path(base path="Path to save txt files", name or relative path=w1398) -> (appended path=w1399:path)
                n769 = flat-sequence {
                  tunnel: w1399 -> [w1403]
                  tunnel: w1398 -> [w1406]
                  tunnel: [w1403] -> w1382
                  tunnel: w1382 -> [w1407]
                  frame #0 {
                    n770 = Build Array(w1406, "" ("Element")) -> (w1405:string[])
                    n771 = call-poly <vilib>:"Write To Spreadsheet File.vi"("1D data"=w1405, "file path (dialog if empty)"=w1403) -> ()  [unwired: 6 in, 1 out]
                  }
                  frame #1 {
                    n772 = local read "Attached Array"() -> (w1409:string[][])
                    n773 = call-poly <vilib>:"Write To Spreadsheet File.vi"("append to file? (new file:F)"=TRUE, "2D data"=w1409, "file path (dialog if empty)"=w1407) -> ()  [unwired: 5 in, 1 out]
                  }
                }
              }
              frame "ED33 reset" {
                n774 = flat-sequence {
                  tunnel: w1418 -> [w1443]
                  frame #0 {
                    w1435 = u32 10000  # timeout (10sec)
                    # "Specified number of bytes is read."
                    # "Note: it can be used by other applications without exiting LabVIEW By closing the serial port."
                    # "Close session with port."
                    # "Serial port is configured (baud rate, data bits, parity, stop bits and flow control)."
                    n775 = local read "Port ED33"() -> (w1421:refnum<visa-resource-name>)
                    n776 = call-poly "VISA Configure Serial Port"("VISA resource name"=w1421, "timeout (10sec)"=w1435, "baud rate (9600)"="baud rate 2", "data bits (8)"="data bits 2", "parity (0:none)"="parity 2", "error in (no error)"=w1443, "stop bits (10: 1 bit)"="stop bits 2", "flow control (0:none)"="flow control 2") -> ("VISA resource name out"=w1440:refnum<visa-resource-name>, "error out"=w1441:errorcluster)  [unwired: 1 in, 5 out]
                    n777 = case shown="True" "write 4" {
                      tunnel: [w1448 w1453] -> w1430
                      tunnel: w1440 -> [w1447 w1452]
                      tunnel: w1441 -> [w1448 w1451]
                      tunnel: [w1447 w1450] -> w1429
                      tunnel: "write 5" -> [_ w1449]
                      frame False {
                      }
                      frame True {
                        # "Send bytes to port."
                        n778 = VISA Write(VISA resource name=w1452, write buffer=w1449, error in (no error)=w1451) -> (VISA resource name out=w1450:refnum<visa-resource-name>, error out=w1453:errorcluster)  [unwired: 1 out]
                      }
                    }
                    n779 = stacked-sequence {
                      tunnel: w1430 -> [w1446]
                      tunnel: [w1446] -> w1424
                      tunnel: w1429 -> [w1445]
                      tunnel: [w1445] -> w1425
                      frame #0 {
                        n780 = Wait (ms)(milliseconds to wait="delay before read (ms) 2") -> ()  [unwired: 1 out]
                      }
                    }
                    n781 = property class="Instr"(reference=w1425, error in=w1424) -> (reference out=w1426:refnum<visa-resource-name>, error out=w1423:errorcluster, "Serial Settings:Number of Bytes at Serial Port"=w1427:u32)
                    "bytes read 2" <- w1427
                    n782 = VISA Read(VISA resource name=w1426, byte count=w1427, error in (no error)=w1423) -> (VISA resource name out=w1438:refnum<visa-resource-name>, read buffer=→"read string 3":string, error out=w1439:errorcluster)  [unwired: 1 out]
                    n783 = VISA Close(VISA resource name=w1438, error in (no error)=w1439) -> (error out=w1437:errorcluster)
                    n784 = call <vilib>:"Simple Error Handler.vi"("error in (no error)"=w1437) -> ()  [unwired: 1 in, 8 out]
                  }
                  frame #1 {
                    n785 = local read "sequence active?"() -> (w1454:bool)
                    n786 = Not(x=w1454) -> (.not. x?=w1455:bool)
                    n787 = case shown="True" w1455 {
                      frame False {
                      }
                      frame True {
                        n788 = local read "KMT read start"() -> (w1456:bool)
                        n789 = case shown="True" w1456 {
                          frame False {
                            n790 = local write "key stm"("ED33" ("key stm")) -> ()
                          }
                          frame True {
                            n791 = local write "key stm"("KMT" ("key stm")) -> ()
                          }
                        }
                      }
                    }
                  }
                }
              }
              frame "Aktuelle Position ED33" {
                n792 = flat-sequence {
                  tunnel: ["wait"] -> w1459
                  frame #0 {
                    w1480 = u32 10000  # timeout (10sec)
                    # "Specified number of bytes is read."
                    # "Note: it can be used by other applications without exiting LabVIEW By closing the serial port."
                    # "Close session with port."
                    n793 = call-poly "VISA Configure Serial Port"("VISA resource name"="VISA-Referenz (Eingang)", "timeout (10sec)"=w1480, "baud rate (9600)"="baud rate 3", "data bits (8)"="data bits 3", "parity (0:none)"="parity 3", "stop bits (10: 1 bit)"="stop bits 3", "flow control (0:none)"="flow control 3") -> ("VISA resource name out"=w1485:refnum<visa-resource-name>, "error out"=w1486:errorcluster)  [unwired: 2 in, 5 out]
                    n794 = case shown="True" "write 6" {
                      tunnel: [w1493 w1498] -> w1475
                      tunnel: w1485 -> [w1492 w1497]
                      tunnel: w1486 -> [w1493 w1496]
                      tunnel: [w1492 w1495] -> w1474
                      tunnel: "write 7" -> [_ w1494]
                      frame False {
                      }
                      frame True {
                        # "Send bytes to port."
                        n795 = VISA Write(VISA resource name=w1497, write buffer=w1494, error in (no error)=w1496) -> (VISA resource name out=w1495:refnum<visa-resource-name>, error out=w1498:errorcluster)  [unwired: 1 out]
                      }
                    }
                    n796 = stacked-sequence {
                      tunnel: w1475 -> [w1491]
                      tunnel: [w1491] -> w1469
                      tunnel: w1474 -> [w1490]
                      tunnel: [w1490] -> w1470
                      frame #0 {
                        n797 = Wait (ms)(milliseconds to wait="delay before read (ms) 3") -> ()  [unwired: 1 out]
                      }
                    }
                    n798 = property class="Instr"(reference=w1470, error in=w1469) -> (reference out=w1471:refnum<visa-resource-name>, error out=w1468:errorcluster, "Serial Settings:Number of Bytes at Serial Port"=w1472:u32)
                    "bytes read 3" <- w1472
                    n799 = VISA Read(VISA resource name=w1471, byte count=w1472, error in (no error)=w1468) -> (VISA resource name out=w1483:refnum<visa-resource-name>, read buffer=w1467:string, error out=w1484:errorcluster)  [unwired: 1 out]
                    n800 = VISA Close(VISA resource name=w1483, error in (no error)=w1484) -> (error out=w1482:errorcluster)
                    n801 = String Subset(string=w1467, offset (0)=9 ("Offset (0)"), length (rest)=8 ("Länge (Rest)")) -> (substring=w1464:string)
                    n802 = call <vilib>:"Simple Error Handler.vi"("error in (no error)"=w1482) -> ()  [unwired: 1 in, 8 out]
                    n803 = Hexadecimal String To Number(string=w1464) -> (number=w1463:u32)  [unwired: 2 in, 1 out]
                    n804 = Number To Decimal String(number=w1463) -> (decimal integer string=w1462:string)  [unwired: 1 in]
                    n805 = local write "Position Y ED33"(w1462) -> ()
                  }
                  frame #1 {
                    n806 = local write "key stm"("auto" ("key stm")) -> ()
                  }
                }
              }
              frame "ED33 Set initial position" {
                n807 = flat-sequence {
                  frame #0 {
                    w1517 = u32 10000  # timeout (10sec)
                    w1544 = u32 10000  # timeout (10sec)
                    # "Specified number of bytes is read."
                    # "Note: it can be used by other applications without exiting LabVIEW By closing the serial port."
                    # "Close session with port."
                    # "Specified number of bytes is read."
                    # "Note: it can be used by other applications without exiting LabVIEW By closing the serial port."
                    # "Close session with port."
                    n808 = call-poly "VISA Configure Serial Port"("VISA resource name"="VISA-Referenz (Eingang) 3", "timeout (10sec)"=w1517, "baud rate (9600)"="baud rate 5", "data bits (8)"="data bits 5", "parity (0:none)"="parity 5", "stop bits (10: 1 bit)"="stop bits 5", "flow control (0:none)"="flow control 5") -> ("VISA resource name out"=w1522:refnum<visa-resource-name>, "error out"=w1523:errorcluster)  [unwired: 2 in, 5 out]
                    n809 = call-poly "VISA Configure Serial Port"("VISA resource name"="VISA-Referenz (Eingang) 2", "timeout (10sec)"=w1544, "baud rate (9600)"="baud rate 4", "data bits (8)"="data bits 4", "parity (0:none)"="parity 4", "stop bits (10: 1 bit)"="stop bits 4", "flow control (0:none)"="flow control 4") -> ("VISA resource name out"=w1549:refnum<visa-resource-name>, "error out"=w1550:errorcluster)  [unwired: 2 in, 5 out]
                    n810 = case shown="True" "write 9" {
                      tunnel: [w1557 w1562] -> w1512
                      tunnel: w1522 -> [w1556 w1561]
                      tunnel: w1523 -> [w1557 w1560]
                      tunnel: [w1556 w1559] -> w1511
                      tunnel: "write 10" -> [_ w1558]
                      frame False {
                      }
                      frame True {
                        # "Send bytes to port."
                        n811 = VISA Write(VISA resource name=w1561, write buffer=w1558, error in (no error)=w1560) -> (VISA resource name out=w1559:refnum<visa-resource-name>, error out=w1562:errorcluster)  [unwired: 1 out]
                      }
                    }
                    n812 = case shown="True" "write 8" {
                      tunnel: [w1567 w1572] -> w1539
                      tunnel: w1549 -> [w1566 w1571]
                      tunnel: w1550 -> [w1567 w1570]
                      tunnel: [w1566 w1569] -> w1538
                      tunnel: "write9" -> [_ w1568]
                      frame False {
                      }
                      frame True {
                        # "Send bytes to port."
                        n813 = VISA Write(VISA resource name=w1571, write buffer=w1568, error in (no error)=w1570) -> (VISA resource name out=w1569:refnum<visa-resource-name>, error out=w1572:errorcluster)  [unwired: 1 out]
                      }
                    }
                    n814 = stacked-sequence {
                      tunnel: w1512 -> [w1555]
                      tunnel: [w1555] -> w1506
                      tunnel: w1511 -> [w1554]
                      tunnel: [w1554] -> w1507
                      frame #0 {
                        n815 = Wait (ms)(milliseconds to wait="delay before read (ms) 5") -> ()  [unwired: 1 out]
                      }
                    }
                    n816 = stacked-sequence {
                      tunnel: w1539 -> [w1565]
                      tunnel: [w1565] -> w1533
                      tunnel: w1538 -> [w1564]
                      tunnel: [w1564] -> w1534
                      frame #0 {
                        n817 = Wait (ms)(milliseconds to wait="delay before read (ms) 4") -> ()  [unwired: 1 out]
                      }
                    }
                    n818 = property class="Instr"(reference=w1507, error in=w1506) -> (reference out=w1508:refnum<visa-resource-name>, error out=w1505:errorcluster, "Serial Settings:Number of Bytes at Serial Port"=w1509:u32)
                    "bytes read 5" <- w1509
                    n819 = property class="Instr"(reference=w1534, error in=w1533) -> (reference out=w1535:refnum<visa-resource-name>, error out=w1532:errorcluster, "Serial Settings:Number of Bytes at Serial Port"=w1536:u32)
                    "bytes read 4" <- w1536
                    n820 = VISA Read(VISA resource name=w1535, byte count=w1536, error in (no error)=w1532) -> (VISA resource name out=w1547:refnum<visa-resource-name>, read buffer=w1531:string, error out=w1548:errorcluster)  [unwired: 1 out]
                    n821 = VISA Close(VISA resource name=w1547, error in (no error)=w1548) -> (error out=w1546:errorcluster)
                    n822 = String Subset(string=w1531, offset (0)=9 ("Offset (0)"), length (rest)=8 ("Länge (Rest)")) -> (substring=w1528:string)
                    n823 = call <vilib>:"Simple Error Handler.vi"("error in (no error)"=w1546) -> ()  [unwired: 1 in, 8 out]
                    n824 = VISA Read(VISA resource name=w1508, byte count=w1509, error in (no error)=w1505) -> (VISA resource name out=w1520:refnum<visa-resource-name>, read buffer=→"read string 4":string, error out=w1521:errorcluster)  [unwired: 1 out]
                    n825 = Hexadecimal String To Number(string=w1528) -> (number=w1527:u32)  [unwired: 2 in, 1 out]
                    n826 = Number To Decimal String(number=w1527) -> (decimal integer string=w1526:string)  [unwired: 1 in]
                    n827 = local write "Position Y ED33 2"(w1526) -> ()
                    n828 = VISA Close(VISA resource name=w1520, error in (no error)=w1521) -> (error out=w1519:errorcluster)
                    n829 = call <vilib>:"Simple Error Handler.vi"("error in (no error)"=w1519) -> ()  [unwired: 1 in, 8 out]
                  }
                  frame #1 {
                    n830 = local write "key stm"("Current position Ed33" ("key stm")) -> ()
                  }
                }
              }
              frame "store data" {
                # "stores the table \"sensor log\" in a file"
                n831 = local read "current sequence"() -> (w1579:string[])
                n832 = local read "sensor log"() -> (w1580:string[][])
                n833 = Array Subset(array=w1579, index=1 ("Index"), length=3) -> (w1578:string[])
                n834 = Build Array (concatenate)(w1578, w1580) -> (w1575:string[][])
                n835 = call-poly <vilib>:"Write To Spreadsheet File.vi"("2D data"=w1575) -> ()  [unwired: 7 in, 1 out]
              }
              frame "Save Array" {
                # "Saves as EXCEL table"
                n836 = invoke on="Attached Array" class="Arr (strikt)" method="Export Data to Excel"(error in=w1586) -> (error out=w1585:errorcluster)  [unwired: 2 in, 2 out]
              }
              frame "Delete Array " {
                n837 = invoke on="Attached Array" class="Arr (strikt)" method="Reinit To Default"(error in=w1590) -> (error out=w1589:errorcluster)  [unwired: 2 in, 2 out]
              }
            }
          }
          frame Error {
            n838 = Unbundle(w1592) -> ("source"=w1595:string)  [unwired: 2 out]
            n839 = One Button Dialog(message=w1595) -> (true=w1594:bool)  [unwired: 1 in]
            n840 = local write "Stopped"(w1594) -> ()
            n841 = local write "stop handover"(w1594) -> ()
          }
        }
        n842 = flat-sequence {
          tunnel: [w237] -> w205
          tunnel: w224 -> [w236]
          frame #0 {
            n843 = local read "key stm"() -> (w238:string)
            n844 = case shown="\"auto\"" w238 {
              selector: w238 -> [w239 _]
              tunnel: [w239 w241] -> w237
              tunnel: w236 -> [_ w241]
              frame "pause", Default {
                n845 = local write "key stm"("auto") -> ()
              }
              frame "auto" {
              }
            }
          }
        }
        n846 = local read "Stopped"() -> (w227:bool)
        "STM run" <- w207
      }
    }
  }
  n847 = local write "error IO"(w1) -> ()
  n848 = call <vilib>:"General Error Handler.vi"("error in (no error)"=w1) -> ()  [unwired: 10 in, 5 out]
